vi "SpatialResolutionAnalysis-3D-8.vi"() -> ()   [LabVIEW 2024]
uses:
  <vilib>/Utility/miscctls.llb/LVBoundsTypeDef.ctl
  <vilib>/Utility/file.llb/Read Delimited Spreadsheet (DBL).vi
  <vilib>/picture/picture.llb/Draw True-Color Pixmap.vi
  <vilib>/gmath/NumericalOptimization/Nonlinear Curve Fit LM.vi
  <vilib>/regexp/Match Regular Expression.xnode
  <vilib>/Analysis/NI_AALBase.lvlib
  <vilib>/vision/NI_Vision_Development_Module.lvlib
  <vilib>/gmath/NI_Gmath.lvlib
panel:
  in  "saved parameter":dbl=15.0 format="%_6g"
  in  "save z pos?":bool
  in  "stop":bool
  in  "Range":cluster{"Lower value":sgl, "Upper value":sgl}={"Lower value"=302.0, "Upper value"=60055.0} {"Upper value" format="%.2f"; "Lower value" format="%.2f"}
  out "Numeric 3":i32=84
  out "profile 3":cluster{dbl[], dbl[]}[](graph)=[{[1.0, 1.0, 1.0, 1.0, 1.0, 1.0, 1.0, 1.0, 1.0, 1.0, 1.0, 1.0, 1.0, 2.0, 2.0, 2.0, 2.0, 2.0, 2.0, 2.0, 2.0, 2.0, 2.0, 2.0, 2.0, 2.0, 2.0, 2.0, 2.0, 2.0, 2.0, 5.0, 5.0, 5.0, 5.0, 5.0, 5.0, 5.0, 5.0, 5.0, 5.0, 5.0, 7.0, 7.0, 7.0, 7.0, 7.0, 7.0, 7.0, 7.0, 7.0, 7.0, 7.0, 7.0, 7.0, 7.0, 7.0, 7.0, 7.0, 7.0, 7.0, 3.0, 3.0, 3.0, 3.0, 3.0, 3.0, 3.0, 3.0, 3.0, 3.0, 1.0, 1.0, 15.0, 15.0, 15.0, 15.0, 15.0, 15.0, 15.0, 15.0, 15.0, 15.0, 15.0], [2.0133468228805937, 1.9830288608829862, 2.1410287615069046, 1.832229816874938, 1.7978233224426952, 1.968242110714196, 1.9933673041983153, 1.724601336050431, 2.5477060719979314, 1.9551201440941726, 1.8397170015620559, 2.236128582607133, 1.6264858204323749, 1.7869746298019815, 1.4196170843904827, 1.5374078182883288, 1.3782496628376637, 1.249895903925542, 1.3942037102048412, 1.4225030278735062, 1.433688545286691, 1.6920898620277007, 1.4435654626803172, 1.5101131998673663, 1.3060720728708268, 1.3178193530013447, 1.3649052519631513, 1.3097046992665182, 1.1134639493452403, 1.4424009490483098, 1.3428675394578506, 0.9421271973201978, 0.9192575100649564, 0.9861704571320219, 0.9992144079023442, 1.0853243609470147, 1.0439557604247962, 0.9041106621598265, 1.018147408083164, 1.1510621119284095, 1.115567444721871, 1.0954616791711456, 0.9694461946565243, 0.8684690878139703, 0.9376717749758984, 0.882216863445789, 1.1744088254801954, 0.9802461660244323, 0.997486368266876, 0.9419455677499634, 0.8628880149840508, 0.9268116414439239, 0.9181180722394033, 0.9776435525722661, 0.988995905088057, 0.9682008357747482, 0.9086257593875379, 1.040188271600828, 0.9299724706944195, 0.950388089905051, 0.9567309022594485, 1.221935897751796, 1.2090462045089128, 1.1438235149609108, 1.1493714387895813, 1.4345461597606564, 1.2239934520828633, 1.090228607115402, 1.354029262137178, 1.1569869611045591, 1.1967020722858934, 1.790272222951798, 1.6210900623548556, 1.0405059212935388, 1.0073358603798341, 0.9444257912585194, 0.9334882181118135, 0.9743355532381182, 0.8814598803657637, 0.8002331400158834, 0.8911247435086341, 0.8792614835678078, 0.921037700924059, 1.103404933894596]}, {[1.0, 1.0, 1.0, 1.0, 1.0, 1.0, 1.0, 1.0, 1.0, 1.0, 1.0, 1.0, 1.0, 2.0, 2.0, 2.0, 2.0, 2.0, 2.0, 2.0, 2.0, 2.0, 2.0, 2.0, 2.0, 2.0, 2.0, 2.0, 2.0, 2.0, 2.0, 5.0, 5.0, 5.0, 5.0, 5.0, 5.0, 5.0, 5.0, 5.0, 5.0, 5.0, 7.0, 7.0, 7.0, 7.0, 7.0, 7.0, 7.0, 7.0, 7.0, 7.0, 7.0, 7.0, 7.0, 7.0, 7.0, 7.0, 7.0, 7.0, 7.0, 3.0, 3.0, 3.0, 3.0, 3.0, 3.0, 3.0, 3.0, 3.0, 3.0, 1.0, 1.0, 15.0, 15.0, 15.0, 15.0, 15.0, 15.0, 15.0, 15.0, 15.0, 15.0, 15.0], [0.5349334014605461, 0.5381337297866883, 0.4325981122029295, 0.48916164520111804, 0.41556148299600454, 0.4850930072283453, 0.5673499365078756, 0.41714778173647393, 0.5526918869297825, 0.4923530041708235, 0.40501938702299484, 0.5082824398122024, 0.40354912909306634, 0.4530438324743144, 0.40779143741716084, 0.43077367983236237, 0.4671352516734954, 0.44629410664345487, 0.43158661278236216, 0.460271541886513, 0.4823249226541753, 0.5185727753496806, 0.4342974192886344, 0.45128050875740255, 0.4303885061603996, 0.5613218585443758, 0.41414445836126024, 0.44047765290288826, 0.47877243294417343, 0.46874740911159807, 0.4766614558480549, 0.4715857966455718, 0.4126072744806765, 0.42646841052591805, 0.40400976642452985, 0.4170504502787077, 0.48205219262233473, 0.41850180617403737, 0.41018388053645777, 0.44390188098962224, 0.41139907883701454, 0.4708303593503039, 0.4344403779325276, 0.46686047747542514, 0.48489083305355846, 0.4497629633492164, 0.46772433252337453, 0.4350416687080472, 0.40360520731331323, 0.4707299669639263, 0.38041949280922327, 0.4546761270737233, 0.44998728304625246, 0.48068592467547, 0.45909266188082487, 0.46566773053329674, 0.429218030475882, 0.41626874590441315, 0.4025480710092228, 0.46728163765248365, 0.46270168477314766, 0.47982606424071567, 0.40715128547570484, 0.4780994379451638, 0.40534745089527735, 0.44748638155411247, 0.49443443713902363, 0.44945698447630245, 0.46059272499696885, 0.43471888991751273, 0.4579720680900581, 0.43868811930073554, 0.4575463738995445, 0.45301271071412846, 0.4456849122856345, 0.44451647252412074, 0.46478062104722645, 0.40834206512347104, 0.46347713941761265, 0.4372934806506643, 0.4423639123216805, 0.4369146593472033, 0.4358778204397408, 0.4152090259272386]}, {[1.0, 1.0, 1.0, 1.0, 1.0, 1.0, 1.0, 1.0, 1.0, 1.0, 1.0, 1.0, 1.0, 2.0, 2.0, 2.0, 2.0, 2.0, 2.0, 2.0, 2.0, 2.0, 2.0, 2.0, 2.0, 2.0, 2.0, 2.0, 2.0, 2.0, 2.0, 5.0, 5.0, 5.0, 5.0, 5.0, 5.0, 5.0, 5.0, 5.0, 5.0, 5.0, 7.0, 7.0, 7.0, 7.0, 7.0, 7.0, 7.0, 7.0, 7.0, 7.0, 7.0, 7.0, 7.0, 7.0, 7.0, 7.0, 7.0, 7.0, 7.0, 3.0, 3.0, 3.0, 3.0, 3.0, 3.0, 3.0, 3.0, 3.0, 3.0, 1.0, 1.0, 15.0, 15.0, 15.0, 15.0, 15.0, 15.0, 15.0, 15.0, 15.0, 15.0, 15.0], [3.831063954171339, 3.059270830960583, 2.2982579267548897, 2.3512738574978624, 2.5538730276997903, 2.682560025330636, 2.6597875381449065, 2.7703141417989587, 3.0330629921976042, 2.546439917288072, 2.6225831316766848, 2.9353823913534747, 2.5991986482523224, 2.9173052067251684, 1.8789100817054876, 2.3734797215792143, 2.697188165514373, 2.0361242582660344, 2.698308173308555, 2.350622719228334, 2.1194094323864903, 2.83503408541773, 2.7683697804028498, 2.30213227302792, 2.8419209826307865, 2.1369921122360855, 2.009733489485215, 2.2188668846287496, 2.560644376786411, 2.0491758147172847, 2.29388213242103, 1.7032091300547687, 2.091295013582046, 1.8883702079287457, 1.5722793767576724, 1.497749085955476, 2.091931566369123, 1.804947152977885, 1.7777195448400112, 1.9539350987425426, 1.7816406998254182, 1.6103878576696868, 2.243284723289365, 1.439263985649626, 1.4421140948685303, 1.6012718104278727, 1.892588797177571, 1.8938395298902209, 1.663961362731013, 1.7664503089155017, 1.5923626379429023, 1.7924631613346518, 1.860054650973308, 1.8546487258879, 1.7533530517676261, 1.6570807100677052, 1.7721806371618676, 1.860204996421116, 1.9831442631444507, 1.7905475389437313, 1.8278060844960526, 2.14740251637709, 1.6527221427498724, 2.2734081810795557, 1.7682142456430505, 2.351440748167282, 2.039692073403972, 2.249697494044236, 2.019669976655679, 2.3817391436774127, 2.1044693016718634, 2.945123441454935, 3.132984030089959, 1.4322347170702565, 1.8617388862479958, 1.7668984450954066, 1.9239338358912674, 1.7440910356590962, 1.8497936230767198, 1.9984535114889663, 1.9016492433228582, 1.8183778696194395, 1.756109772929477, 1.864696210002186]}, {[1.0, 1.0, 1.0, 1.0, 1.0, 1.0, 1.0, 1.0, 1.0, 1.0, 1.0, 1.0, 1.0, 2.0, 2.0, 2.0, 2.0, 2.0, 2.0, 2.0, 2.0, 2.0, 2.0, 2.0, 2.0, 2.0, 2.0, 2.0, 2.0, 2.0, 2.0, 5.0, 5.0, 5.0, 5.0, 5.0, 5.0, 5.0, 5.0, 5.0, 5.0, 5.0, 7.0, 7.0, 7.0, 7.0, 7.0, 7.0, 7.0, 7.0, 7.0, 7.0, 7.0, 7.0, 7.0, 7.0, 7.0, 7.0, 7.0, 7.0, 7.0, 3.0, 3.0, 3.0, 3.0, 3.0, 3.0, 3.0, 3.0, 3.0, 3.0, 1.0, 1.0, 15.0, 15.0, 15.0, 15.0, 15.0, 15.0, 15.0, 15.0, 15.0, 15.0, 15.0], [2.1950609171334663, 2.054618641938806, 2.104623270933475, 2.175230158941747, 1.8063966644943987, 2.1295671490810504, 2.209023498381645, 2.0515957222532695, 2.9990312250832534, 2.2759668684117713, 2.281844375004091, 2.4517643206281377, 0.9998405968995983, 1.9895569035078806, 1.386277332900748, 1.477211472520211, 1.4491295731261742, 1.295484538599624, 1.2209490171797608, 1.328049693706136, 1.3871687988938963, 1.6950226848823489, 1.3919183622385123, 1.530122363720778, 1.4218506232848938, 1.814696520405228, 1.499546890762415, 1.3528630093363747, 1.1830279345524057, 1.4487275307919036, 1.3903221708836062, 0.9299541953106812, 0.8839351063390566, 1.035489598307442, 1.009482788308503, 1.054044052714303, 1.0236198842257271, 1.0318268251460063, 1.1225026575045192, 1.167009429834893, 0.9257403035306736, 1.070234933121553, 0.9920706919584273, 0.9140544351981513, 0.8757808606546661, 0.8718346074707618, 1.0110444436389308, 0.9520818427957021, 0.9768177701203681, 0.9915186544650038, 0.9230083868636685, 0.9046033708789486, 0.9099211724070002, 1.002151816664439, 0.9608485679370016, 0.9125676936610334, 0.9660386410221703, 1.078401400423473, 1.0023703508557482, 0.895286648365859, 0.9716597443982098, 1.1949613429126829, 1.161748827048745, 1.1631282077159188, 1.148313006075648, 1.3735217290054094, 1.2433597954356586, 1.1662345174848958, 1.2701690085899722, 1.1727390746235637, 1.1971761228612998, 2.0031359293798054, 2.0609983678438337, 0.9149174421733332, 1.0525064576834762, 0.9347056385035375, 0.946629434078085, 1.5404013619903427, 0.930605986788623, 0.9051875232044269, 0.894279488961371, 0.8718853102409165, 0.9292096538995072, 1.0776975442315762]}, {[1.0, 1.0, 1.0, 1.0, 1.0, 1.0, 1.0, 1.0, 1.0, 1.0, 1.0, 1.0, 1.0, 2.0, 2.0, 2.0, 2.0, 2.0, 2.0, 2.0, 2.0, 2.0, 2.0, 2.0, 2.0, 2.0, 2.0, 2.0, 2.0, 2.0, 2.0, 5.0, 5.0, 5.0, 5.0, 5.0, 5.0, 5.0, 5.0, 5.0, 5.0, 5.0, 7.0, 7.0, 7.0, 7.0, 7.0, 7.0, 7.0, 7.0, 7.0, 7.0, 7.0, 7.0, 7.0, 7.0, 7.0, 7.0, 7.0, 7.0, 7.0, 3.0, 3.0, 3.0, 3.0, 3.0, 3.0, 3.0, 3.0, 3.0, 3.0, 1.0, 1.0, 15.0, 15.0, 15.0, 15.0, 15.0, 15.0, 15.0, 15.0, 15.0, 15.0, 15.0], [2.9152156827594293, 2.5990526581184956, 1.906401812221069, 2.3686457243679144, 2.121321629827777, 2.3179713514009026, 2.392123629004429, 2.3037200675462755, 2.9146261263558007, 2.0648914087567856, 2.484756888015519, 2.4235500991471604, 1.533300131698492, 2.500295338025416, 2.3348778310327094, 2.405355608068957, 2.528663329870978, 2.2469147380725674, 2.4434672372828383, 2.1118260376977456, 2.721672790630798, 3.1052449674871614, 2.7801574803549274, 2.627964587450267, 2.474809806384693, 1.7158461369035183, 2.1448277490061587, 2.0290842777452047, 2.463419621353616, 3.5693252371416606, 2.5104117383774973, 2.241237982322342, 1.7078526466721193, 2.0495685256164693, 1.7370219820601127, 1.8245896378450086, 2.5086646334752323, 2.1859796911332667, 2.180925068929074, 2.012040182338204, 2.273553445872903, 1.949240216124691, 2.5350823425047007, 1.573081961156342, 1.867172753412812, 2.141389794448718, 2.0778586256984615, 2.0938614883880526, 2.101194097948842, 1.992923549444901, 1.7936881545636807, 1.9749097104449778, 2.045208462819868, 2.2293085556006202, 2.2248086215455687, 2.1608335627654767, 2.262287525483442, 2.2543964739278, 2.0932173803022063, 2.0184068032417786, 2.150789163948129, 2.2053407496814255, 2.106580809562779, 2.0176046290868026, 2.104550211229832, 2.4659027742456647, 2.2702529865700116, 2.284568939068995, 2.2528486161897474, 2.268035269102454, 2.2830606744651365, 2.8430238588896906, 2.8219479955311835, 1.7946822327277403, 2.334201107146507, 2.032573581439689, 2.183270787877003, 2.124268915381388, 1.9879932478731197, 2.344731423243975, 2.0123274416218733, 2.215117623104961, 2.2701610476768646, 2.247837372716093]}]
  out "Image":T1(plugin-control)
  out "obj index":i32
  in  "analysis file":path=path "E:/PSFvsR.anal"
  in  "delete":bool
  in  "add":bool
  in  "stocked object index":i32(slide) min=0 max=2 scale=0.0..2.0
  in  "stocked / raw":bool=TRUE
  out "FWHMx'":dbl=1.1390586789611326
  out "FWHMz'":dbl=2.7153633068041123
  out "x'":cluster{dbl[], dbl[]}[](graph)=[{[-2.1729316492173996, -1.9681427393245199, -1.7633538294316402, -1.5585649195387605, -1.353776009645881, -1.1489870997530014, -0.9441981898601217, -0.739409279967242, -0.5346203700743624, -0.32983146018148274, -0.1250425502886031, 0.07974635960427658, 0.28453526949715624, 0.48932417939003586, 0.6941130892829155, 0.8989019991757952, 1.1036909090686748, 1.3084798189615545, 1.5132687288544342, 1.7180576387473139, 1.9228465486401933], [49.0, 26.0, 15.0, 15.0, 19.0, 38.0, 88.0, 186.0, 324.0, 487.0, 578.0, 545.0, 450.0, 335.0, 242.0, 169.0, 120.0, 87.0, 69.0, 57.0, 47.0]}, {array[1000 elements], array[1000 elements]}]
  out "z'":cluster{dbl[], dbl[]}[](graph)=[{[-2.9476850843070337, -2.742896174414154, -2.5381072645212743, -2.333318354628395, -2.128529444735515, -1.9237405348426353, -1.7189516249497558, -1.5141627150568762, -1.3093738051639965, -1.1045848952711168, -0.8997959853782371, -0.6950070754853575, -0.49021816559247783, -0.2854292556995982, -0.08064034580671856, 0.1241485640861611, 0.3289374739790408, 0.5337263838719204, 0.7385152937648001, 0.9433042036576798, 1.1480931135505594, 1.352882023443439, 1.5576709333363186, 1.7624598432291982, 1.967248753122078, 2.1720376630149576, 2.376826572907837], [33.0, 39.0, 53.0, 72.0, 93.0, 128.0, 182.0, 228.0, 282.0, 342.0, 407.0, 503.0, 557.0, 578.0, 538.0, 507.0, 494.0, 456.0, 415.0, 378.0, 329.0, 274.0, 240.0, 223.0, 188.0, 156.0, 130.0]}, {array[1000 elements], array[1000 elements]}]
  in  "Angle (degrees)":dbl=-23.0 format="%.2f"
  in  "nx'":i32=10
  in  "nz'":i32=13
  out "zx 2":u16[][](graph)=[[0, 0, 0, 0, 0, 0, 214, 195, 168, 154, 142, 125, 111, 106, 109, 112, 114, 112, 109, 111, 116, 122, 126, 126, 124, 124, 134, 0, 0, 0, 0, 0, 0, 0, 0, 0, 0, 0, 0, 0], [0, 0, 0, 0, 0, 0, 234, 188, 163, 151, 142, 128, 115, 115, 114, 113, 112, 112, 112, 113, 119, 125, 127, 126, 128, 133, 135, 134, 127, 0, 0, 0, 0, 0, 0, 0, 0, 0, 0, 0], [0, 0, 0, 0, 0, 246, 230, 176, 154, 145, 128, 122, 119, 118, 117, 115, 113, 113, 116, 117, 121, 128, 130, 135, 146, 153, 152, 138, 125, 122, 124, 0, 0, 0, 0, 0, 0, 0, 0, 0], [0, 0, 0, 0, 0, 215, 201, 171, 153, 138, 128, 123, 121, 120, 118, 115, 114, 112, 111, 118, 125, 132, 138, 153, 168, 169, 153, 141, 131, 128, 126, 117, 113, 114, 0, 0, 0, 0, 0, 0], [0, 0, 0, 0, 257, 240, 191, 168, 146, 132, 128, 126, 124, 122, 118, 116, 115, 113, 112, 121, 131, 133, 145, 162, 170, 162, 150, 142, 137, 136, 133, 119, 114, 116, 111, 105, 0, 0, 0, 0], [0, 0, 0, 0, 279, 243, 192, 163, 140, 126, 125, 126, 123, 119, 116, 116, 115, 117, 122, 127, 134, 139, 148, 164, 171, 161, 155, 149, 149, 145, 135, 123, 119, 118, 114, 104, 106, 108, 0, 0], [0, 0, 0, 274, 280, 223, 182, 157, 136, 124, 121, 122, 119, 116, 114, 114, 114, 122, 133, 138, 146, 153, 160, 171, 179, 177, 165, 155, 155, 148, 135, 129, 128, 127, 121, 113, 109, 108, 105, 104], [0, 0, 0, 259, 246, 198, 164, 150, 138, 132, 128, 123, 119, 116, 116, 116, 115, 121, 135, 149, 162, 172, 182, 181, 190, 191, 177, 164, 158, 148, 139, 135, 133, 127, 121, 115, 112, 111, 107, 106], [0, 0, 0, 243, 225, 184, 157, 148, 143, 141, 138, 127, 117, 117, 115, 117, 118, 123, 130, 146, 169, 193, 206, 207, 208, 206, 187, 177, 168, 155, 143, 137, 128, 120, 115, 113, 112, 113, 108, 109], [0, 0, 217, 224, 214, 179, 167, 157, 147, 148, 147, 137, 126, 118, 114, 114, 117, 124, 128, 155, 195, 228, 243, 250, 242, 221, 198, 185, 176, 162, 146, 135, 124, 118, 113, 109, 111, 113, 113, 114], [0, 0, 190, 203, 199, 187, 176, 164, 155, 160, 159, 150, 134, 118, 112, 110, 112, 124, 147, 186, 238, 282, 295, 294, 271, 239, 207, 190, 181, 169, 150, 133, 126, 122, 114, 111, 112, 115, 116, 115], [0, 161, 169, 188, 185, 190, 186, 173, 164, 166, 166, 157, 135, 116, 113, 112, 114, 135, 168, 216, 279, 328, 340, 325, 292, 251, 216, 193, 187, 174, 150, 135, 129, 124, 117, 116, 118, 119, 118, 115], [0, 149, 162, 174, 176, 184, 188, 178, 170, 166, 168, 157, 132, 113, 111, 116, 125, 147, 188, 250, 327, 382, 388, 354, 303, 259, 221, 206, 198, 181, 154, 139, 131, 126, 123, 120, 121, 122, 119, 116], [133, 137, 156, 167, 169, 179, 187, 183, 176, 174, 173, 160, 134, 118, 113, 116, 128, 157, 216, 298, 384, 442, 441, 390, 329, 282, 248, 226, 207, 184, 163, 149, 137, 133, 130, 126, 126, 125, 119, 119], [127, 132, 145, 157, 162, 177, 196, 190, 181, 183, 183, 166, 141, 124, 117, 119, 133, 166, 238, 337, 442, 507, 506, 449, 373, 315, 276, 236, 204, 181, 164, 151, 140, 137, 133, 131, 132, 126, 118, 113], [123, 126, 137, 146, 155, 172, 193, 191, 178, 184, 193, 169, 140, 124, 119, 123, 141, 182, 257, 373, 509, 603, 578, 496, 403, 326, 276, 234, 198, 174, 158, 145, 139, 137, 134, 131, 129, 122, 115, 112], [117, 122, 132, 139, 149, 175, 185, 177, 173, 180, 183, 163, 133, 115, 116, 122, 138, 185, 264, 407, 574, 657, 617, 527, 427, 333, 267, 223, 189, 170, 153, 143, 138, 135, 132, 125, 121, 120, 118, 115], [118, 121, 125, 132, 146, 166, 175, 166, 163, 174, 171, 149, 126, 115, 115, 119, 138, 188, 286, 424, 587, 678, 645, 550, 435, 342, 269, 220, 187, 169, 157, 147, 138, 132, 127, 121, 122, 124, 121, 116], [122, 120, 121, 129, 139, 152, 159, 157, 158, 164, 157, 135, 120, 117, 120, 123, 143, 201, 298, 422, 550, 638, 631, 536, 420, 337, 276, 221, 186, 165, 157, 148, 137, 129, 125, 125, 129, 131, 124, 117], [125, 123, 122, 128, 133, 142, 147, 146, 153, 156, 143, 124, 112, 115, 116, 123, 143, 186, 284, 408, 536, 607, 594, 512, 416, 336, 271, 219, 183, 158, 145, 142, 137, 131, 129, 134, 138, 135, 127, 123], [126, 123, 123, 128, 140, 147, 146, 141, 146, 141, 140, 126, 116, 114, 117, 127, 145, 185, 270, 389, 517, 594, 577, 503, 406, 316, 251, 206, 177, 157, 142, 135, 130, 127, 130, 134, 139, 136, 133, 132], [123, 120, 120, 126, 139, 145, 147, 144, 147, 151, 144, 129, 117, 117, 123, 133, 149, 189, 267, 373, 488, 556, 553, 484, 384, 291, 229, 189, 169, 155, 140, 130, 123, 124, 128, 135, 138, 139, 141, 140], [121, 122, 123, 121, 125, 135, 136, 138, 147, 148, 139, 125, 118, 121, 127, 137, 154, 192, 255, 357, 464, 515, 504, 442, 348, 272, 215, 180, 163, 152, 138, 127, 123, 127, 137, 141, 143, 149, 151, 148], [121, 124, 126, 123, 125, 132, 134, 135, 138, 135, 129, 119, 119, 124, 127, 137, 151, 180, 235, 328, 428, 478, 465, 415, 337, 262, 203, 177, 160, 147, 136, 129, 129, 137, 147, 147, 151, 159, 159, 153], [121, 123, 126, 123, 124, 130, 133, 134, 132, 130, 125, 122, 122, 123, 123, 134, 148, 173, 223, 304, 383, 429, 430, 390, 317, 242, 195, 173, 155, 142, 137, 132, 136, 141, 143, 146, 153, 158, 159, 154], [126, 130, 131, 129, 127, 129, 133, 133, 128, 129, 127, 121, 121, 122, 130, 140, 152, 173, 211, 268, 332, 374, 393, 359, 285, 216, 180, 161, 148, 140, 139, 136, 136, 138, 138, 144, 152, 164, 165, 163], [131, 136, 134, 130, 128, 132, 136, 128, 120, 124, 124, 120, 121, 125, 137, 146, 154, 168, 194, 235, 289, 340, 367, 342, 273, 198, 157, 147, 141, 140, 140, 137, 135, 136, 140, 151, 169, 179, 174, 172], [124, 127, 128, 128, 130, 133, 135, 126, 120, 123, 120, 118, 121, 127, 137, 145, 151, 162, 180, 213, 270, 323, 349, 337, 268, 197, 156, 143, 136, 138, 141, 141, 137, 135, 143, 163, 182, 184, 178, 0], [116, 122, 127, 132, 133, 134, 134, 129, 126, 126, 124, 122, 125, 131, 141, 149, 154, 156, 168, 204, 250, 288, 309, 314, 250, 190, 160, 145, 134, 134, 138, 139, 135, 139, 149, 170, 184, 185, 185, 0], [117, 120, 126, 135, 131, 135, 137, 135, 132, 130, 129, 128, 133, 142, 149, 157, 159, 154, 163, 193, 230, 256, 267, 258, 221, 181, 160, 144, 131, 125, 130, 130, 129, 135, 150, 165, 177, 183, 0, 0], [118, 119, 123, 129, 130, 135, 140, 139, 136, 134, 130, 129, 135, 142, 148, 153, 154, 150, 155, 177, 208, 230, 244, 226, 199, 175, 158, 140, 130, 124, 125, 126, 127, 137, 150, 167, 186, 184, 0, 0], [118, 122, 126, 124, 130, 138, 139, 135, 135, 135, 126, 125, 134, 142, 142, 144, 146, 141, 146, 165, 187, 208, 225, 218, 200, 177, 150, 139, 131, 126, 124, 124, 128, 137, 154, 181, 198, 0, 0, 0], [108, 117, 118, 120, 128, 138, 136, 132, 132, 130, 125, 124, 132, 138, 141, 141, 140, 135, 141, 157, 172, 186, 203, 207, 190, 161, 143, 135, 129, 125, 125, 123, 126, 139, 160, 185, 197, 0, 0, 0], [105, 109, 113, 117, 125, 130, 131, 129, 129, 128, 123, 118, 123, 133, 138, 136, 133, 128, 133, 144, 159, 173, 189, 200, 180, 149, 140, 136, 130, 128, 131, 133, 138, 148, 164, 178, 185, 0, 0, 0], [0, 0, 113, 110, 101, 117, 120, 122, 123, 121, 116, 113, 119, 130, 134, 126, 126, 124, 124, 139, 155, 167, 180, 188, 175, 151, 142, 138, 133, 136, 141, 143, 146, 149, 161, 170, 0, 0, 0, 0], [0, 0, 0, 0, 101, 110, 106, 116, 120, 116, 110, 110, 116, 122, 120, 117, 120, 121, 121, 134, 148, 159, 169, 178, 168, 153, 145, 142, 141, 144, 147, 142, 146, 151, 164, 167, 0, 0, 0, 0], [0, 0, 0, 0, 0, 0, 109, 116, 118, 113, 109, 105, 110, 112, 110, 110, 114, 116, 119, 128, 140, 152, 160, 165, 159, 152, 148, 143, 148, 154, 149, 144, 145, 153, 164, 0, 0, 0, 0, 0], [0, 0, 0, 0, 0, 0, 0, 0, 0, 111, 108, 107, 105, 106, 106, 109, 112, 110, 113, 123, 135, 145, 150, 152, 152, 152, 151, 151, 152, 152, 148, 144, 142, 151, 154, 0, 0, 0, 0, 0], [0, 0, 0, 0, 0, 0, 0, 0, 0, 0, 0, 108, 96, 95, 102, 109, 110, 109, 113, 123, 132, 137, 137, 138, 147, 158, 165, 163, 160, 160, 153, 146, 145, 153, 0, 0, 0, 0, 0, 0], [0, 0, 0, 0, 0, 0, 0, 0, 0, 0, 0, 0, 0, 96, 103, 110, 111, 111, 116, 120, 125, 126, 127, 132, 146, 164, 174, 169, 166, 169, 164, 151, 148, 153, 0, 0, 0, 0, 0, 0]]
  out "num of points":i32=3
  out "profile 2":cluster{dbl[], dbl[]}[](graph)=[{[15.0, 15.0, 15.0], [0.8792614835678078, 0.921037700924059, 1.103404933894596]}, {[15.0, 15.0, 15.0], [0.4369146593472033, 0.4358778204397408, 0.4152090259272386]}, {[15.0, 15.0, 15.0], [1.8183778696194395, 1.756109772929477, 1.864696210002186]}, {[15.0, 15.0, 15.0], [0.8718853102409165, 0.9292096538995072, 1.0776975442315762]}, {[15.0, 15.0, 15.0], [2.215117623104961, 2.2701610476768646, 2.247837372716093]}]
  out "z [um]":dbl=0.23987999999999998
  out "Nx":i32=109
  out "Ny":i32=57
  out "Nz":i32=40
  out "z ofst and pixsize":dbl[](array[numeric])=[0.57912, 0.20475]
  in  "most recent":bool=TRUE
  in  "folderpath":path=path "E:/20241006-215727beads"
  out "Numeric 2":i32=2402
  in  "fitting range y":dbl=8.0
  in  "fitting range z":dbl=30.0
  out "Particle Reports (Pixels)":T2(array[cluster])=[{"Area"=37.0, "Number of Holes"=0.0, "Bounding Rect"={"Left"=52.0, "Top"=2.0, "Right"=63.0, "Bottom"=7.0}, "Center of Mass"={"X"=57.16216216216216, "Y"=3.6216216216216215}, "Orientation"=179.34423482631453, "Dimensions"={"Width"=11.0, "Height"=5.0}}, {"Area"=30.0, "Number of Holes"=0.0, "Bounding Rect"={"Left"=29.0, "Top"=4.0, "Right"=44.0, "Bottom"=9.0}, "Center of Mass"={"X"=36.166666666666664, "Y"=5.733333333333333}, "Orientation"=165.68755166285754, "Dimensions"={"Width"=15.0, "Height"=5.0}}, {"Area"=8.0, "Number of Holes"=0.0, "Bounding Rect"={"Left"=76.0, "Top"=5.0, "Right"=81.0, "Bottom"=7.0}, "Center of Mass"={"X"=78.0, "Y"=5.625}, "Orientation"=-0.0, "Dimensions"={"Width"=5.0, "Height"=2.0}}, {"Area"=6.0, "Number of Holes"=0.0, "Bounding Rect"={"Left"=90.0, "Top"=5.0, "Right"=94.0, "Bottom"=7.0}, "Center of Mass"={"X"=91.5, "Y"=5.333333333333333}, "Orientation"=-0.0, "Dimensions"={"Width"=4.0, "Height"=2.0}}, {"Area"=1.0, "Number of Holes"=0.0, "Bounding Rect"={"Left"=22.0, "Top"=6.0, "Right"=23.0, "Bottom"=7.0}, "Center of Mass"={"X"=22.0, "Y"=6.0}, "Orientation"=-0.0, "Dimensions"={"Width"=1.0, "Height"=1.0}}, {"Area"=9.0, "Number of Holes"=0.0, "Bounding Rect"={"Left"=67.0, "Top"=6.0, "Right"=72.0, "Bottom"=9.0}, "Center of Mass"={"X"=69.33333333333333, "Y"=7.222222222222222}, "Orientation"=167.962250872462, "Dimensions"={"Width"=5.0, "Height"=3.0}}, {"Area"=10.0, "Number of Holes"=0.0, "Bounding Rect"={"Left"=82.0, "Top"=11.0, "Right"=87.0, "Bottom"=13.0}, "Center of Mass"={"X"=84.0, "Y"=11.5}, "Orientation"=-0.0, "Dimensions"={"Width"=5.0, "Height"=2.0}}, {"Area"=7.0, "Number of Holes"=0.0, "Bounding Rect"={"Left"=92.0, "Top"=11.0, "Right"=97.0, "Bottom"=13.0}, "Center of Mass"={"X"=94.14285714285714, "Y"=11.285714285714286}, "Orientation"=175.69217590792118, "Dimensions"={"Width"=5.0, "Height"=2.0}}, {"Area"=6.0, "Number of Holes"=0.0, "Bounding Rect"={"Left"=65.0, "Top"=13.0, "Right"=69.0, "Bottom"=15.0}, "Center of Mass"={"X"=66.83333333333333, "Y"=13.333333333333334}, "Orientation"=167.06682160295298, "Dimensions"={"Width"=4.0, "Height"=2.0}}, {"Area"=7.0, "Number of Holes"=0.0, "Bounding Rect"={"Left"=73.0, "Top"=13.0, "Right"=77.0, "Bottom"=15.0}, "Center of Mass"={"X"=74.28571428571429, "Y"=13.571428571428571}, "Orientation"=171.65037788300214, "Dimensions"={"Width"=4.0, "Height"=2.0}}, {"Area"=24.0, "Number of Holes"=0.0, "Bounding Rect"={"Left"=22.0, "Top"=14.0, "Right"=32.0, "Bottom"=18.0}, "Center of Mass"={"X"=27.0, "Y"=15.625}, "Orientation"=14.883749397417526, "Dimensions"={"Width"=10.0, "Height"=4.0}}, {"Area"=24.0, "Number of Holes"=0.0, "Bounding Rect"={"Left"=48.0, "Top"=15.0, "Right"=55.0, "Bottom"=21.0}, "Center of Mass"={"X"=51.041666666666664, "Y"=17.541666666666668}, "Orientation"=140.81219786217568, "Dimensions"={"Width"=7.0, "Height"=6.0}}, {"Area"=15.0, "Number of Holes"=0.0, "Bounding Rect"={"Left"=10.0, "Top"=19.0, "Right"=15.0, "Bottom"=23.0}, "Center of Mass"={"X"=12.333333333333334, "Y"=20.266666666666666}, "Orientation"=174.11585553399107, "Dimensions"={"Width"=5.0, "Height"=4.0}}, {"Area"=8.0, "Number of Holes"=0.0, "Bounding Rect"={"Left"=29.0, "Top"=20.0, "Right"=34.0, "Bottom"=23.0}, "Center of Mass"={"X"=31.25, "Y"=21.125}, "Orientation"=164.64358614242056, "Dimensions"={"Width"=5.0, "Height"=3.0}}, {"Area"=6.0, "Number of Holes"=0.0, "Bounding Rect"={"Left"=77.0, "Top"=21.0, "Right"=81.0, "Bottom"=23.0}, "Center of Mass"={"X"=78.5, "Y"=21.333333333333332}, "Orientation"=-0.0, "Dimensions"={"Width"=4.0, "Height"=2.0}}, {"Area"=12.0, "Number of Holes"=0.0, "Bounding Rect"={"Left"=26.0, "Top"=25.0, "Right"=30.0, "Bottom"=30.0}, "Center of Mass"={"X"=27.833333333333332, "Y"=26.833333333333332}, "Orientation"=69.54280838998545, "Dimensions"={"Width"=4.0, "Height"=5.0}}, {"Area"=3.0, "Number of Holes"=0.0, "Bounding Rect"={"Left"=70.0, "Top"=26.0, "Right"=73.0, "Bottom"=27.0}, "Center of Mass"={"X"=71.0, "Y"=26.0}, "Orientation"=-0.0, "Dimensions"={"Width"=3.0, "Height"=1.0}}, {"Area"=7.0, "Number of Holes"=0.0, "Bounding Rect"={"Left"=4.0, "Top"=28.0, "Right"=8.0, "Bottom"=30.0}, "Center of Mass"={"X"=5.714285714285714, "Y"=28.428571428571427}, "Orientation"=171.65037788300342, "Dimensions"={"Width"=4.0, "Height"=2.0}}, {"Area"=5.0, "Number of Holes"=0.0, "Bounding Rect"={"Left"=83.0, "Top"=28.0, "Right"=86.0, "Bottom"=30.0}, "Center of Mass"={"X"=84.2, "Y"=28.4}, "Orientation"=161.56505117709622, "Dimensions"={"Width"=3.0, "Height"=2.0}}, {"Area"=9.0, "Number of Holes"=0.0, "Bounding Rect"={"Left"=89.0, "Top"=28.0, "Right"=94.0, "Bottom"=30.0}, "Center of Mass"={"X"=91.22222222222223, "Y"=28.444444444444443}, "Orientation"=175.26883889599605, "Dimensions"={"Width"=5.0, "Height"=2.0}}, {"Area"=7.0, "Number of Holes"=0.0, "Bounding Rect"={"Left"=52.0, "Top"=29.0, "Right"=57.0, "Bottom"=31.0}, "Center of Mass"={"X"=53.857142857142854, "Y"=29.714285714285715}, "Orientation"=175.6921759079141, "Dimensions"={"Width"=5.0, "Height"=2.0}}, {"Area"=7.0, "Number of Holes"=0.0, "Bounding Rect"={"Left"=65.0, "Top"=29.0, "Right"=69.0, "Bottom"=31.0}, "Center of Mass"={"X"=66.71428571428571, "Y"=29.428571428571427}, "Orientation"=171.65037788300276, "Dimensions"={"Width"=4.0, "Height"=2.0}}, {"Area"=1.0, "Number of Holes"=0.0, "Bounding Rect"={"Left"=96.0, "Top"=29.0, "Right"=97.0, "Bottom"=30.0}, "Center of Mass"={"X"=96.0, "Y"=29.0}, "Orientation"=-0.0, "Dimensions"={"Width"=1.0, "Height"=1.0}}, {"Area"=25.0, "Number of Holes"=0.0, "Bounding Rect"={"Left"=3.0, "Top"=33.0, "Right"=9.0, "Bottom"=38.0}, "Center of Mass"={"X"=5.4, "Y"=34.96}, "Orientation"=10.870389527236576, "Dimensions"={"Width"=6.0, "Height"=5.0}}, {"Area"=16.0, "Number of Holes"=0.0, "Bounding Rect"={"Left"=59.0, "Top"=33.0, "Right"=65.0, "Bottom"=36.0}, "Center of Mass"={"X"=61.75, "Y"=33.875}, "Orientation"=172.42714692778492, "Dimensions"={"Width"=6.0, "Height"=3.0}}, {"Area"=1.0, "Number of Holes"=0.0, "Bounding Rect"={"Left"=25.0, "Top"=34.0, "Right"=26.0, "Bottom"=35.0}, "Center of Mass"={"X"=25.0, "Y"=34.0}, "Orientation"=-0.0, "Dimensions"={"Width"=1.0, "Height"=1.0}}, {"Area"=9.0, "Number of Holes"=0.0, "Bounding Rect"={"Left"=39.0, "Top"=40.0, "Right"=44.0, "Bottom"=42.0}, "Center of Mass"={"X"=41.22222222222222, "Y"=40.44444444444444}, "Orientation"=175.26883889598594, "Dimensions"={"Width"=5.0, "Height"=2.0}}, {"Area"=1.0, "Number of Holes"=0.0, "Bounding Rect"={"Left"=73.0, "Top"=42.0, "Right"=74.0, "Bottom"=43.0}, "Center of Mass"={"X"=73.0, "Y"=42.0}, "Orientation"=-0.0, "Dimensions"={"Width"=1.0, "Height"=1.0}}, {"Area"=8.0, "Number of Holes"=0.0, "Bounding Rect"={"Left"=35.0, "Top"=43.0, "Right"=39.0, "Bottom"=45.0}, "Center of Mass"={"X"=36.5, "Y"=43.5}, "Orientation"=-0.0, "Dimensions"={"Width"=4.0, "Height"=2.0}}, {"Area"=8.0, "Number of Holes"=0.0, "Bounding Rect"={"Left"=30.0, "Top"=44.0, "Right"=34.0, "Bottom"=46.0}, "Center of Mass"={"X"=31.5, "Y"=44.5}, "Orientation"=-0.0, "Dimensions"={"Width"=4.0, "Height"=2.0}}, {"Area"=2.0, "Number of Holes"=0.0, "Bounding Rect"={"Left"=53.0, "Top"=44.0, "Right"=55.0, "Bottom"=45.0}, "Center of Mass"={"X"=53.5, "Y"=44.0}, "Orientation"=-0.0, "Dimensions"={"Width"=2.0, "Height"=1.0}}, {"Area"=36.0, "Number of Holes"=0.0, "Bounding Rect"={"Left"=36.0, "Top"=46.0, "Right"=47.0, "Bottom"=51.0}, "Center of Mass"={"X"=40.52777777777778, "Y"=47.77777777777778}, "Orientation"=171.22278809294195, "Dimensions"={"Width"=11.0, "Height"=5.0}}, {"Area"=5.0, "Number of Holes"=0.0, "Bounding Rect"={"Left"=88.0, "Top"=46.0, "Right"=91.0, "Bottom"=48.0}, "Center of Mass"={"X"=89.2, "Y"=46.6}, "Orientation"=18.4349488228699, "Dimensions"={"Width"=3.0, "Height"=2.0}}, {"Area"=8.0, "Number of Holes"=0.0, "Bounding Rect"={"Left"=74.0, "Top"=48.0, "Right"=79.0, "Bottom"=51.0}, "Center of Mass"={"X"=76.5, "Y"=48.875}, "Orientation"=7.545786339297439, "Dimensions"={"Width"=5.0, "Height"=3.0}}, {"Area"=3.0, "Number of Holes"=0.0, "Bounding Rect"={"Left"=48.0, "Top"=50.0, "Right"=51.0, "Bottom"=51.0}, "Center of Mass"={"X"=49.0, "Y"=50.0}, "Orientation"=-0.0, "Dimensions"={"Width"=3.0, "Height"=1.0}}, {"Area"=30.0, "Number of Holes"=0.0, "Bounding Rect"={"Left"=66.0, "Top"=51.0, "Right"=77.0, "Bottom"=55.0}, "Center of Mass"={"X"=71.83333333333333, "Y"=52.833333333333336}, "Orientation"=4.05699723021086, "Dimensions"={"Width"=11.0, "Height"=4.0}}, {"Area"=4.0, "Number of Holes"=0.0, "Bounding Rect"={"Left"=83.0, "Top"=52.0, "Right"=86.0, "Bottom"=54.0}, "Center of Mass"={"X"=84.0, "Y"=52.25}, "Orientation"=-0.0, "Dimensions"={"Width"=3.0, "Height"=2.0}}, {"Area"=4.0, "Number of Holes"=0.0, "Bounding Rect"={"Left"=35.0, "Top"=54.0, "Right"=39.0, "Bottom"=55.0}, "Center of Mass"={"X"=36.5, "Y"=54.0}, "Orientation"=-0.0, "Dimensions"={"Width"=4.0, "Height"=1.0}}, {"Area"=2.0, "Number of Holes"=0.0, "Bounding Rect"={"Left"=99.0, "Top"=55.0, "Right"=101.0, "Bottom"=56.0}, "Center of Mass"={"X"=99.5, "Y"=55.0}, "Orientation"=-0.0, "Dimensions"={"Width"=2.0, "Height"=1.0}}]
  out "error z":dbl=0.6513882337485863
  out "error y":dbl=3.612958681902941
  out "error x":dbl=1.7215369706106136
  out "file path (use dialog)":path=path "E:/20241006-215727beads/20241006-215727beadsaiviatif/20241006-215727beads_t0.aivia.tif"
  out "yx 5":u16[][](graph)=[[135, 135, 135, 135, 135, 135, 135, 135, 135, 135, 135, 135, 135, 135, 135, 135, 135, 135, 135, 135], [135, 135, 135, 135, 135, 135, 135, 135, 135, 136, 135, 135, 135, 135, 135, 135, 135, 135, 135, 135], [135, 135, 135, 135, 135, 135, 135, 135, 136, 138, 138, 138, 136, 135, 135, 135, 135, 135, 135, 135], [135, 135, 135, 135, 135, 135, 135, 136, 139, 143, 145, 142, 138, 136, 135, 135, 135, 135, 135, 135], [135, 135, 135, 135, 135, 135, 135, 138, 145, 155, 160, 154, 144, 138, 135, 135, 135, 135, 135, 135], [135, 135, 135, 135, 135, 135, 135, 141, 156, 177, 186, 174, 154, 141, 136, 135, 135, 135, 135, 135], [135, 135, 135, 135, 135, 135, 136, 146, 173, 211, 228, 207, 169, 145, 137, 135, 135, 135, 135, 135], [135, 135, 135, 135, 135, 135, 138, 153, 197, 258, 287, 252, 190, 151, 138, 135, 135, 135, 135, 135], [135, 135, 135, 135, 135, 135, 139, 161, 222, 313, 355, 302, 214, 157, 139, 135, 135, 135, 135, 135], [135, 135, 135, 135, 135, 135, 140, 167, 245, 362, 418, 349, 233, 163, 139, 135, 135, 135, 135, 135], [135, 135, 135, 135, 135, 136, 141, 171, 258, 390, 455, 377, 245, 165, 139, 135, 135, 135, 135, 135], [135, 135, 135, 135, 135, 136, 142, 172, 259, 387, 451, 376, 247, 166, 140, 135, 135, 135, 135, 135], [135, 135, 135, 135, 135, 135, 142, 170, 245, 357, 412, 348, 236, 163, 139, 135, 135, 135, 135, 135], [135, 135, 135, 135, 135, 135, 140, 163, 222, 308, 351, 303, 215, 158, 138, 135, 135, 135, 135, 135], [135, 135, 135, 135, 135, 135, 138, 154, 196, 256, 284, 252, 191, 152, 137, 135, 135, 135, 135, 135], [135, 135, 135, 135, 135, 135, 137, 147, 173, 209, 227, 207, 170, 145, 136, 135, 135, 135, 135, 135], [135, 135, 135, 135, 135, 135, 136, 142, 156, 175, 185, 174, 154, 140, 135, 135, 135, 135, 135, 135], [135, 135, 135, 135, 135, 135, 135, 138, 145, 154, 159, 154, 144, 137, 135, 135, 135, 135, 135, 135], [135, 135, 135, 135, 135, 135, 135, 136, 139, 143, 145, 143, 139, 136, 135, 135, 135, 135, 135, 135], [135, 135, 135, 135, 135, 135, 135, 135, 136, 138, 138, 138, 136, 135, 135, 135, 135, 135, 135, 135]]
  out "yx 4":u16[][](graph)=[[134, 132, 133, 133, 131, 134, 137, 129, 132, 138, 137, 132, 131, 134, 131, 132, 135, 133, 134, 132], [139, 137, 134, 132, 128, 131, 135, 137, 141, 132, 130, 136, 134, 127, 128, 135, 136, 133, 133, 136], [139, 135, 133, 129, 129, 132, 137, 140, 137, 136, 134, 134, 144, 144, 145, 137, 133, 133, 129, 132], [137, 135, 143, 138, 134, 130, 135, 141, 137, 129, 135, 136, 141, 140, 133, 128, 129, 127, 123, 126], [135, 138, 148, 151, 151, 144, 146, 141, 126, 119, 143, 148, 145, 135, 130, 127, 129, 126, 124, 130], [134, 134, 141, 146, 155, 147, 146, 144, 137, 132, 143, 161, 157, 137, 134, 135, 129, 127, 125, 129], [136, 138, 138, 134, 146, 143, 137, 140, 143, 140, 204, 249, 191, 141, 132, 137, 129, 126, 127, 126], [134, 137, 141, 140, 157, 153, 145, 137, 138, 220, 372, 326, 212, 151, 135, 134, 129, 130, 130, 122], [137, 138, 140, 135, 146, 158, 152, 153, 187, 287, 384, 308, 172, 144, 134, 134, 140, 131, 128, 126], [144, 145, 142, 131, 141, 149, 144, 189, 262, 389, 467, 337, 176, 139, 134, 138, 136, 130, 125, 135], [139, 141, 141, 136, 136, 141, 158, 235, 350, 389, 460, 371, 188, 136, 126, 137, 131, 130, 132, 139], [132, 136, 138, 134, 129, 152, 174, 238, 274, 350, 459, 372, 199, 139, 135, 137, 133, 132, 133, 133], [131, 135, 140, 142, 146, 166, 194, 211, 242, 298, 382, 363, 227, 143, 140, 137, 130, 131, 127, 131], [132, 131, 141, 143, 146, 164, 184, 208, 230, 257, 345, 384, 236, 154, 136, 137, 134, 135, 134, 128], [127, 125, 142, 142, 144, 160, 176, 188, 188, 229, 277, 273, 201, 146, 134, 132, 132, 131, 137, 127], [126, 126, 139, 145, 150, 153, 157, 165, 176, 191, 203, 223, 179, 146, 134, 126, 125, 130, 140, 134], [126, 128, 139, 143, 144, 149, 148, 150, 158, 181, 215, 216, 176, 147, 127, 123, 130, 133, 138, 138], [125, 129, 137, 137, 132, 144, 145, 142, 148, 165, 178, 180, 170, 140, 125, 128, 133, 131, 131, 131], [127, 135, 136, 136, 133, 145, 148, 147, 151, 152, 153, 156, 149, 131, 128, 130, 130, 129, 100, 57], [123, 131, 133, 132, 129, 136, 134, 132, 134, 127, 139, 156, 143, 129, 130, 127, 127, 96, 31, 0]]
  out "tilt 3":dbl=-2.58289224144748
  out "tilt 2":dbl=-0.0
  out "yx 3":dbl[][](graph)=[[134.9499399241804, 134.94993992735928, 134.94994011666108, 134.94994689756712, 134.9500925508678, 134.95195835824072, 134.96606856510073, 135.02781171692624, 135.17711556967282, 135.35038463951318, 135.37644338631844, 135.2244142667145, 135.0566683599304, 134.97501589369142, 134.95349979728468, 134.9502452829951, 134.94995575067753, 134.94994041978086, 134.94993993352654, 134.94993992425526], [134.9499399242392, 134.94993993335143, 134.94994048551243, 134.94996061318204, 134.9504006417102, 134.95613902239515, 135.00033887194684, 135.1975188179371, 135.6848005274849, 136.26787953279342, 136.37812751009096, 135.88507467377178, 135.31990636868235, 135.03838011568922, 134.96271419768144, 134.95105478828853, 134.94999871461098, 134.94994179737762, 134.94993996021208, 134.94993992456756], [134.9499399243755, 134.94993994751263, 134.94994137413596, 134.94999429541951, 134.95117181943053, 134.96680457262556, 135.08944178243138, 135.6471792762914, 137.05557441999412, 138.79216924098975, 139.1862015556717, 137.7720988416936, 136.08594260181818, 135.22623709815605, 134.99054428971715, 134.95354544667816, 134.95013337154785, 134.9499461954365, 134.94994004699086, 134.94993992560194], [134.9499399246508, 134.9499399766896, 134.94994324170767, 134.9500664949676, 134.95285767123644, 134.9905805974951, 135.29197712506408, 136.68928195160558, 140.2943015429152, 144.87209202520933, 146.0804514174922, 142.49432006079542, 138.03974585043812, 135.71454651806232, 135.06426567821296, 134.96026871083725, 134.95050376136743, 134.94995852176808, 134.94994029479477, 134.9499399286114], [134.94993992513238, 134.94994002880847, 134.9499466478417, 134.95020091934956, 134.95606140258818, 135.0366918898231, 135.69279059897846, 138.79340481913627, 146.9654860105327, 157.64667072832867, 160.85486247623967, 152.81483574912534, 142.39413724374913, 136.82421988875507, 135.23507473891496, 134.9761498161115, 134.95139564938893, 134.94998877732283, 134.9499409147641, 134.94993993628518], [134.94993992585512, 134.9499401088182, 134.94995199483336, 134.95041664734075, 134.96131619259967, 135.11397343522592, 136.3790462064828, 142.4730198216657, 158.8790208441416, 180.93910878077205, 188.35523286759542, 172.4224030399425, 150.83684784044036, 139.01967101628068, 135.5798684105343, 135.00885358099595, 134.9532691243449, 134.95005359864493, 134.94994226937763, 134.94993995338328], [134.94993992677044, 134.94994021278094, 134.9499591192651, 134.9507112446351, 134.9686673534806, 135.22467914697657, 137.38529540200508, 147.99371367830858, 177.1626612565863, 217.4933948282034, 232.47610173976352, 204.57391598322062, 164.98273190369258, 142.77759703368173, 136.18266740194838, 135.067240881991, 134.95668419865305, 134.95017422189753, 134.9499448422802, 134.94993998652603], [134.94993992771643, 134.94994032375197, 134.94996696276223, 134.95104537205142, 134.97724801441615, 135.35754874851784, 138.62610515879672, 154.9829250269071, 200.9121974656826, 266.1833916769077, 292.70844833509454, 249.53822746968171, 185.24054551190682, 148.28615834582135, 137.08680810677933, 135.15682157054144, 134.96204215389344, 134.9503676918799, 134.94994906001668, 134.9499400420418], [134.94993992844917, 134.9499404142072, 134.94997366164986, 134.95134330815011, 134.9852126741441, 135.48561484892466, 139.8653812079921, 162.2034789879957, 226.25240402236568, 319.76667293534297, 360.9972158488822, 302.00378062405514, 209.54547788534947, 155.07644810248232, 138.23106825076442, 135.27314427366477, 134.9691766154357, 134.95063172764435, 134.94995495675587, 134.94994012151983], [134.9499399287403, 134.94994045650395, 134.94997721276198, 134.9515180789105, 134.99029722741122, 135.57352237519683, 140.77184110307024, 167.7923464492414, 246.89484023274008, 365.50404198157094, 421.8565748548583, 350.67844211616676, 232.96067873012018, 161.85531161044693, 139.41269987928794, 135.39720733685098, 134.9770250080548, 134.95093096672227, 134.94996183471605, 134.94994021684226], [134.94993992849118, 134.94994043640807, 134.94997643100024, 134.95151194204726, 134.99084147582073, 135.5929551842416, 141.05798134930382, 170.0075144708553, 256.5296089893872, 389.71463620222283, 457.5145618765073, 381.72054110319846, 249.01937827205404, 166.8098382563467, 140.32667534700894, 135.49820697311725, 134.983720326872, 134.95119750726576, 134.9499682125082, 134.94994030863182], [134.9499399277865, 134.94994036077816, 134.94997158388938, 134.95132699999905, 134.9866590435521, 135.53727170643032, 140.6263523990655, 168.09841752653173, 251.91399794815555, 384.31779281506203, 456.188523741524, 384.9926156643361, 252.54789534583398, 168.36825911489854, 140.6880467984346, 135.54526182704842, 134.9872592928021, 134.95135348956995, 134.94997227582044, 134.9499403715282], [134.94993992684806, 134.9499402538122, 134.9499642447973, 134.95102404516157, 134.97913970274232, 135.4251444331188, 139.62277814467214, 162.7138185076788, 234.62321436824195, 351.1603067109318, 418.33274806566635, 359.3741389882056, 242.34024265108616, 165.99980001957445, 140.37436140417114, 135.5225334124144, 134.98646058106442, 134.95134736436037, 134.94997269747478, 134.94994038526414], [134.94993992592282, 134.9499401446257, 134.94995647337814, 134.950690492316, 134.9705083799166, 135.29051466181093, 138.35733406876116, 155.54824628152502, 210.18839196260438, 301.0031932604985, 356.38894633390987, 313.37672805424427, 221.8190134711307, 160.5045653869426, 139.49221100179582, 135.43777809191963, 134.98159750329054, 134.9511812300633, 134.94996933307283, 134.9499403451447], [134.94993992518144, 134.9499400547628, 134.94994989920195, 134.9504002203048, 134.96277382392358, 135.1661515967061, 137.15083241008162, 148.48679306481972, 185.257795483346, 247.91732907184903, 288.22432283313475, 260.6065268611577, 197.19431924159687, 153.57999849674306, 138.31914540355606, 135.3181027838093, 134.97424805969266, 134.95090968025312, 134.94996330027695, 134.94994026462038], [134.94993992468102, 134.94993999268974, 134.94994524998094, 134.95018996984396, 134.957033258436, 135.07152511186666, 136.20918456216842, 142.83016730799508, 164.74653139327864, 203.02587605732356, 228.92656753752044, 213.33716461279698, 174.45656392892576, 146.98071889707984, 137.1636297824914, 135.19605544413935, 134.9664732576074, 134.95061101458074, 134.94995638305036, 134.94994016805256], [134.94993992439154, 134.9499399560085, 134.94994244295364, 134.95006024371096, 134.95341270228673, 135.0105042699609, 135.58813907275237, 139.01338701012077, 150.58257519548158, 171.2886059332258, 185.9892697964509, 178.2651220948289, 157.16126791004353, 141.8318358970998, 136.2383107445387, 135.09567794087377, 134.9599009491106, 134.9503512958373, 134.9499501892666, 134.94994007892015], [134.94993992424656, 134.94993993726652, 134.94994097935242, 134.94999120886175, 134.95144597098445, 134.97666310920044, 135.2364481915343, 136.8059712244634, 142.21488996082928, 152.13215560075128, 159.50408959311955, 156.15159816719995, 146.01143827606762, 138.43698279352918, 135.6141413637186, 135.02638359552378, 134.95525589339, 134.95016329298372, 134.94994559517744, 134.94994001114426], [134.94993992418335, 134.94993992893268, 134.9499403157216, 134.9499592872286, 134.95051846595143, 134.9603845824188, 135.06387381369134, 135.7008895595083, 137.94060580442965, 142.14648714791187, 145.4135045626645, 144.14245480887547, 139.82958484153738, 136.51503706220902, 135.25325470367568, 134.98545764144671, 134.9524529428354, 134.95004735909862, 134.9499426993504, 134.94993996746348], [134.94993992415925, 134.94993992569383, 134.9499400528618, 134.9499463999834, 134.95013678793697, 134.953555979578, 134.99007309897698, 135.21907552736644, 136.04047085432785, 137.6198954094083, 138.89968668772067, 138.48041932174903, 136.8567055293293, 135.57218309032115, 135.07263359499544, 134.9645577701783, 134.95099223440712, 134.94998569652057, 134.94994112713866, 134.94993994325185]]
  out "yx 2":u16[][](graph)=[[131, 129, 135, 132, 132, 139, 137, 122, 139, 139, 137, 129, 133, 135, 129, 136, 135, 133, 135, 131], [138, 136, 137, 132, 126, 133, 136, 137, 144, 125, 134, 139, 132, 123, 130, 141, 134, 133, 133, 145], [141, 137, 127, 128, 130, 136, 140, 141, 136, 137, 134, 135, 152, 146, 152, 130, 134, 134, 123, 128], [138, 128, 144, 130, 130, 126, 137, 144, 136, 127, 139, 136, 143, 138, 126, 125, 130, 122, 121, 130], [137, 144, 153, 150, 148, 141, 148, 139, 121, 118, 152, 148, 145, 131, 131, 128, 131, 127, 126, 134], [133, 132, 146, 154, 161, 146, 149, 144, 136, 131, 147, 167, 157, 133, 136, 139, 126, 127, 125, 129], [137, 138, 137, 130, 145, 140, 136, 142, 144, 138, 219, 263, 181, 134, 131, 138, 129, 125, 130, 125], [136, 139, 143, 142, 163, 151, 143, 135, 136, 232, 399, 322, 200, 147, 135, 134, 129, 134, 131, 119], [132, 135, 140, 138, 149, 161, 154, 150, 186, 294, 392, 300, 157, 142, 134, 135, 146, 129, 126, 132], [145, 146, 141, 129, 142, 152, 142, 186, 259, 394, 472, 336, 174, 138, 134, 140, 133, 130, 124, 140], [144, 144, 144, 138, 140, 139, 155, 233, 355, 389, 462, 378, 192, 136, 124, 137, 131, 130, 138, 139], [134, 136, 138, 132, 123, 148, 167, 240, 272, 344, 465, 384, 205, 140, 138, 138, 135, 134, 131, 129], [129, 136, 140, 142, 144, 163, 195, 208, 238, 289, 380, 379, 240, 145, 141, 138, 129, 131, 125, 133], [135, 134, 140, 144, 145, 163, 181, 206, 230, 244, 332, 409, 251, 160, 135, 138, 137, 138, 142, 125], [131, 122, 144, 143, 138, 158, 176, 193, 182, 218, 275, 277, 209, 147, 135, 131, 131, 124, 139, 129], [126, 121, 137, 144, 150, 153, 157, 165, 173, 192, 191, 231, 186, 150, 137, 126, 123, 129, 144, 139], [130, 127, 139, 145, 148, 151, 149, 150, 155, 169, 212, 228, 185, 155, 128, 119, 133, 133, 135, 138], [123, 119, 136, 143, 127, 142, 146, 142, 143, 160, 177, 175, 180, 147, 124, 128, 134, 131, 128, 127], [126, 140, 134, 143, 130, 143, 154, 146, 153, 152, 152, 153, 156, 131, 128, 131, 129, 130, 129, 0], [117, 131, 131, 137, 126, 134, 139, 129, 138, 130, 124, 158, 154, 128, 133, 128, 123, 132, 0, 0]]
  out "Numeric":i32=38
  out "#function calls":i32=18
  out "residue":dbl=513.1920909975838
  in  "anal method":T3(ring)
  in  "tilt":dbl=20.0 format="%#_13g"
  in  "indexing variable":i32
  out "Z":i32=16
  out "FWHMz":T4(graph)={"X Values"=[0.49091547409651104, 0.5436936843186253, 0.5964718945407396, 0.6492501047628538, 0.7020283149849681, 0.7548065252070824, 0.8075847354291966, 0.8603629456513109, 0.9131411558734251, 0.9659193660955394, 1.0186975763176538, 1.0714757865397682, 1.1242539967618825, 1.177032206983997, 1.2298104172061113, 1.2825886274282257, 1.33536683765034, 1.3881450478724544, 1.4409232580945688, 1.4937014683166832, 1.5464796785387975, 1.599257888760912, 1.6520360989830263, 1.7048143092051407, 1.757592519427255, 1.8103707296493694, 1.8631489398714838, 1.9159271500935982, 1.9687053603157125, 2.0214835705378267, 2.074261780759941, 2.1270399909820554, 2.17981820120417, 2.232596411426284, 2.2853746216483986, 2.338152831870513, 2.3909310420926273, 2.4437092523147417, 2.496487462536856, 2.5492656727589704, 2.602043882981085, 2.654822093203199, 2.7076003034253135, 2.760378513647428, 2.8131567238695423, 2.8659349340916567, 2.918713144313771, 2.9714913545358854, 3.024269564758, 3.077047774980114], "Histogram: h(x)"=[1, 0, 1, 1, 0, 0, 1, 0, 0, 1, 0, 2, 1, 0, 0, 1, 2, 0, 0, 2, 1, 0, 0, 2, 8, 1, 1, 2, 1, 1, 1, 2, 2, 0, 0, 0, 0, 0, 0, 0, 1, 0, 0, 0, 0, 0, 2, 0, 0, 1]}
  out "FWHMy":T4(graph)={"X Values"=[0.38574742692294495, 0.39994402150286423, 0.4141406160827835, 0.4283372106627028, 0.4425338052426221, 0.4567303998225414, 0.47092699440246066, 0.48512358898237995, 0.49932018356229924, 0.5135167781422185, 0.5277133727221378, 0.5419099673020571, 0.5561065618819764, 0.5703031564618957, 0.584499751041815, 0.5986963456217342, 0.6128929402016535, 0.6270895347815728, 0.6412861293614921, 0.6554827239414114, 0.6696793185213307, 0.68387591310125, 0.6980725076811692, 0.7122691022610885, 0.7264656968410078, 0.7406622914209271, 0.7548588860008464, 0.7690554805807657, 0.783252075160685, 0.7974486697406042, 0.8116452643205235, 0.8258418589004428, 0.8400384534803621, 0.8542350480602814, 0.8684316426402007, 0.88262823722012, 0.8968248318000392, 0.9110214263799585, 0.9252180209598778, 0.9394146155397971, 0.9536112101197164, 0.9678078046996357, 0.982004399279555, 0.9962009938594742, 1.0103975884393934, 1.0245941830193126, 1.0387907775992318, 1.052987372179151, 1.0671839667590701, 1.0813805613389893], "Histogram: h(x)"=[2, 2, 3, 8, 1, 5, 5, 2, 3, 1, 1, 0, 0, 1, 1, 0, 2, 0, 0, 0, 0, 0, 0, 0, 0, 0, 0, 0, 1, 0, 0, 0, 0, 0, 0, 0, 0, 0, 0, 0, 0, 0, 0, 0, 0, 0, 0, 0, 0, 1]}
  out "FWHMx":T4(graph)={"X Values"=[0.038327908101687, 0.114983724305061, 0.191639540508435, 0.26829535671180904, 0.34495117291518307, 0.4216069891185571, 0.4982628053219311, 0.5749186215253052, 0.6515744377286792, 0.7282302539320532, 0.8048860701354272, 0.8815418863388013, 0.9581977025421753, 1.0348535187455492, 1.1115093349489231, 1.188165151152297, 1.264820967355671, 1.3414767835590449, 1.4181325997624188, 1.4947884159657927, 1.5714442321691666, 1.6481000483725405, 1.7247558645759145, 1.8014116807792884, 1.8780674969826623, 1.9547233131860362, 2.03137912938941, 2.108034945592784, 2.184690761796158, 2.261346577999532, 2.338002394202906, 2.4146582104062797, 2.4913140266096536, 2.5679698428130275, 2.6446256590164015, 2.7212814752197754, 2.7979372914231493, 2.874593107626523, 2.951248923829897, 3.027904740033271, 3.104560556236645, 3.181216372440019, 3.257872188643393, 3.3345280048467667, 3.4111838210501406, 3.4878396372535145, 3.5644954534568885, 3.6411512696602624, 3.7178070858636363, 3.79446290206701], "Histogram: h(x)"=[1, 0, 0, 0, 0, 0, 0, 0, 2, 3, 4, 8, 6, 4, 1, 2, 1, 1, 0, 2, 0, 0, 1, 0, 0, 0, 0, 1, 0, 0, 0, 0, 0, 0, 0, 0, 0, 0, 0, 0, 0, 0, 0, 0, 0, 0, 0, 1, 0, 1]}
  in  "intervals":i32=50
  out "FWHMz [um]":dbl=1.894751855635071
  out "xz MIP":i32[][](graph)
  out "zy":u16[][](graph)=[[116, 118, 110, 138, 128, 114, 112, 101, 106, 102, 107, 97, 98, 94, 107, 101, 98, 95, 103, 100, 103, 98, 96, 96, 99, 96, 99, 104, 92, 91, 95, 97, 94, 108, 87, 102, 95, 93, 95, 94], [119, 124, 132, 144, 140, 124, 120, 113, 117, 110, 114, 102, 108, 103, 106, 104, 107, 102, 101, 100, 109, 106, 101, 103, 99, 100, 104, 107, 97, 97, 105, 103, 96, 105, 93, 105, 103, 100, 98, 98], [122, 130, 146, 154, 142, 131, 129, 121, 118, 110, 116, 106, 109, 107, 106, 102, 110, 102, 99, 98, 107, 106, 102, 103, 101, 104, 101, 105, 99, 101, 107, 99, 98, 103, 96, 101, 102, 100, 98, 100], [126, 135, 156, 168, 146, 146, 139, 124, 120, 111, 114, 108, 104, 109, 106, 97, 103, 102, 104, 104, 108, 105, 103, 99, 102, 104, 102, 105, 99, 102, 103, 98, 100, 107, 99, 103, 104, 102, 100, 100], [130, 137, 156, 178, 160, 155, 138, 122, 122, 113, 108, 103, 101, 105, 104, 91, 98, 107, 108, 112, 108, 107, 106, 99, 104, 102, 105, 107, 106, 102, 98, 105, 102, 109, 105, 105, 105, 101, 101, 98], [131, 146, 174, 188, 173, 160, 151, 134, 127, 122, 110, 110, 113, 109, 111, 99, 104, 105, 104, 109, 104, 105, 102, 104, 105, 103, 105, 107, 109, 108, 105, 109, 104, 103, 106, 104, 97, 102, 105, 100], [127, 144, 191, 195, 195, 171, 155, 140, 132, 125, 115, 116, 112, 105, 111, 104, 106, 108, 104, 108, 110, 108, 104, 105, 109, 103, 103, 106, 108, 108, 109, 109, 105, 102, 103, 100, 96, 106, 105, 102], [130, 148, 199, 220, 211, 185, 170, 150, 135, 125, 119, 118, 107, 104, 104, 102, 106, 115, 111, 111, 115, 115, 111, 101, 112, 103, 99, 106, 110, 110, 111, 114, 107, 104, 102, 104, 103, 102, 102, 98], [136, 162, 218, 248, 238, 216, 183, 159, 142, 129, 120, 114, 107, 106, 106, 103, 104, 112, 111, 111, 117, 115, 112, 97, 110, 103, 102, 102, 107, 109, 110, 115, 111, 107, 105, 109, 105, 102, 102, 98], [142, 171, 233, 264, 271, 245, 194, 163, 144, 132, 120, 111, 108, 107, 110, 107, 107, 111, 110, 111, 117, 114, 113, 99, 104, 105, 103, 101, 106, 109, 111, 117, 114, 109, 107, 111, 108, 104, 101, 102], [151, 178, 232, 275, 306, 283, 208, 160, 139, 134, 120, 108, 109, 110, 112, 109, 112, 115, 112, 115, 115, 115, 113, 105, 103, 105, 104, 102, 107, 109, 113, 114, 114, 110, 110, 108, 108, 105, 104, 107], [169, 195, 242, 290, 339, 323, 226, 151, 134, 126, 118, 107, 113, 113, 113, 109, 120, 120, 116, 116, 118, 119, 111, 110, 107, 105, 107, 105, 107, 110, 112, 114, 115, 109, 113, 105, 106, 106, 111, 113], [179, 214, 258, 316, 385, 374, 243, 146, 132, 113, 112, 102, 112, 108, 113, 103, 115, 117, 129, 125, 122, 125, 110, 107, 110, 106, 111, 105, 102, 113, 114, 122, 123, 111, 113, 101, 113, 103, 112, 109], [196, 240, 271, 349, 469, 437, 250, 147, 124, 110, 108, 106, 106, 103, 108, 99, 108, 117, 131, 133, 118, 121, 104, 105, 112, 106, 110, 105, 108, 117, 122, 128, 130, 116, 109, 103, 121, 104, 110, 105], [232, 266, 287, 387, 554, 509, 252, 141, 117, 115, 107, 116, 111, 105, 107, 102, 111, 129, 117, 129, 110, 118, 100, 102, 116, 109, 105, 107, 113, 117, 132, 133, 127, 116, 117, 113, 118, 104, 115, 115], [240, 272, 314, 422, 623, 567, 255, 137, 130, 114, 104, 115, 112, 106, 111, 106, 113, 125, 126, 136, 123, 123, 106, 109, 116, 118, 109, 111, 114, 126, 141, 146, 129, 112, 118, 112, 120, 109, 122, 126], [252, 259, 318, 458, 696, 578, 273, 147, 143, 114, 115, 112, 112, 105, 114, 111, 117, 123, 132, 139, 128, 124, 112, 109, 117, 114, 114, 115, 112, 132, 154, 152, 143, 118, 123, 112, 120, 115, 124, 121], [246, 257, 310, 461, 678, 563, 299, 170, 143, 118, 111, 108, 113, 110, 115, 118, 120, 128, 141, 141, 130, 120, 122, 111, 120, 120, 116, 113, 117, 131, 165, 158, 150, 125, 129, 121, 121, 119, 130, 124], [223, 252, 305, 421, 600, 551, 315, 187, 143, 119, 114, 114, 115, 113, 117, 116, 121, 127, 146, 148, 132, 124, 119, 113, 118, 122, 115, 113, 116, 133, 174, 175, 152, 128, 130, 128, 124, 118, 125, 123], [202, 231, 291, 394, 555, 542, 325, 208, 148, 120, 115, 115, 114, 111, 117, 114, 115, 129, 145, 151, 145, 131, 123, 116, 112, 118, 116, 118, 110, 136, 187, 188, 155, 129, 135, 130, 125, 121, 126, 119], [191, 210, 251, 347, 490, 497, 314, 231, 156, 128, 117, 113, 114, 110, 120, 118, 110, 128, 139, 147, 150, 135, 120, 120, 108, 114, 116, 118, 104, 138, 199, 197, 156, 133, 135, 130, 126, 123, 130, 114], [182, 191, 208, 297, 417, 432, 287, 229, 161, 134, 130, 118, 116, 112, 116, 127, 115, 127, 135, 144, 153, 145, 114, 108, 111, 119, 114, 117, 107, 141, 198, 222, 167, 142, 142, 135, 128, 125, 130, 113], [164, 171, 185, 254, 355, 352, 258, 214, 172, 137, 127, 121, 114, 113, 111, 114, 130, 139, 141, 158, 156, 140, 119, 114, 112, 120, 120, 118, 113, 157, 236, 253, 178, 148, 154, 148, 130, 134, 132, 126], [154, 160, 169, 222, 282, 295, 228, 179, 175, 147, 128, 120, 113, 114, 113, 110, 134, 147, 146, 170, 159, 147, 118, 117, 111, 113, 121, 114, 120, 177, 266, 273, 184, 160, 157, 152, 137, 140, 128, 127], [151, 147, 164, 201, 236, 234, 196, 171, 163, 149, 131, 117, 117, 116, 115, 120, 139, 151, 146, 166, 157, 156, 115, 115, 107, 110, 114, 114, 130, 194, 289, 284, 196, 172, 154, 157, 154, 147, 132, 120], [152, 144, 156, 182, 205, 193, 180, 170, 161, 149, 136, 123, 120, 119, 119, 127, 146, 147, 147, 162, 168, 164, 116, 111, 107, 111, 119, 118, 145, 217, 310, 281, 199, 181, 152, 157, 164, 147, 137, 121], [150, 147, 148, 168, 179, 164, 162, 160, 157, 150, 138, 123, 120, 121, 121, 128, 146, 141, 149, 160, 177, 165, 123, 112, 112, 114, 122, 121, 165, 247, 324, 277, 217, 197, 163, 161, 163, 150, 141, 124], [151, 145, 144, 156, 163, 150, 150, 150, 147, 145, 135, 123, 123, 124, 124, 133, 146, 142, 149, 170, 190, 164, 128, 118, 117, 118, 124, 129, 196, 273, 329, 282, 253, 213, 180, 171, 165, 152, 143, 125], [169, 159, 144, 132, 156, 149, 140, 140, 144, 137, 138, 133, 130, 134, 134, 150, 153, 146, 146, 181, 204, 161, 126, 119, 117, 117, 122, 145, 221, 291, 350, 294, 272, 215, 197, 191, 171, 154, 148, 129], [180, 175, 142, 139, 156, 143, 132, 134, 142, 145, 158, 143, 143, 139, 136, 145, 158, 152, 146, 192, 213, 164, 130, 117, 119, 117, 131, 168, 232, 303, 344, 310, 273, 233, 198, 185, 164, 158, 149, 134], [193, 171, 143, 145, 161, 143, 131, 132, 146, 148, 161, 148, 136, 143, 136, 141, 161, 152, 154, 204, 224, 167, 129, 114, 115, 126, 132, 192, 250, 335, 342, 336, 291, 233, 208, 179, 182, 168, 149, 127], [192, 167, 149, 142, 152, 147, 128, 136, 147, 160, 157, 143, 137, 154, 153, 147, 159, 159, 176, 196, 231, 167, 138, 124, 128, 131, 138, 178, 230, 298, 274, 313, 288, 239, 203, 194, 205, 172, 149, 128], [200, 160, 147, 144, 143, 144, 128, 144, 148, 156, 150, 148, 148, 159, 164, 156, 155, 165, 198, 209, 234, 165, 146, 128, 133, 128, 144, 170, 209, 250, 234, 274, 256, 241, 215, 213, 196, 165, 153, 127], [216, 153, 142, 142, 140, 134, 128, 142, 144, 142, 152, 146, 152, 162, 164, 158, 154, 178, 213, 232, 228, 172, 152, 133, 136, 130, 146, 165, 192, 203, 216, 241, 236, 236, 227, 225, 193, 161, 154, 124], [231, 150, 136, 140, 138, 127, 125, 133, 136, 132, 148, 136, 150, 158, 157, 155, 156, 199, 215, 238, 216, 180, 151, 135, 136, 128, 148, 151, 174, 172, 190, 210, 221, 215, 220, 224, 209, 159, 146, 122], [224, 148, 125, 132, 135, 127, 123, 127, 132, 129, 132, 124, 137, 142, 140, 143, 153, 193, 203, 205, 198, 172, 143, 134, 128, 129, 143, 139, 156, 154, 157, 182, 197, 186, 193, 217, 211, 154, 139, 124], [199, 145, 121, 128, 124, 112, 111, 113, 122, 119, 120, 119, 123, 124, 124, 130, 135, 172, 168, 175, 177, 155, 132, 126, 121, 129, 134, 129, 132, 140, 139, 159, 163, 171, 186, 224, 202, 152, 128, 116], [158, 131, 116, 119, 113, 106, 107, 106, 113, 111, 113, 114, 110, 115, 118, 121, 121, 146, 133, 150, 153, 137, 122, 118, 117, 127, 126, 124, 117, 129, 131, 139, 144, 158, 174, 208, 168, 134, 114, 109], [131, 116, 112, 114, 110, 107, 107, 108, 111, 111, 114, 117, 109, 108, 113, 116, 109, 123, 125, 133, 133, 125, 117, 114, 114, 114, 118, 122, 117, 123, 125, 126, 132, 135, 158, 172, 143, 115, 105, 105], [104, 95, 98, 98, 94, 90, 91, 94, 97, 98, 98, 102, 101, 96, 99, 99, 94, 102, 108, 110, 111, 105, 102, 99, 99, 100, 98, 100, 102, 104, 104, 104, 105, 107, 117, 123, 104, 90, 92, 94]]
  out "zx":u16[][](graph)=[[0, 0, 114, 104, 112, 118, 122, 117, 103, 97, 108, 117, 114, 121, 126, 126, 124, 124, 135, 135, 128, 120, 125, 123, 114, 112, 117, 110, 103, 106, 108, 105, 104, 106, 99, 95, 94, 109, 109, 110], [0, 145, 129, 118, 118, 119, 121, 116, 110, 104, 107, 111, 114, 121, 126, 127, 124, 138, 152, 156, 140, 130, 131, 134, 121, 116, 118, 121, 116, 110, 111, 110, 107, 107, 105, 102, 104, 109, 108, 109], [146, 146, 138, 129, 125, 122, 117, 114, 115, 116, 109, 109, 112, 121, 127, 129, 135, 157, 172, 152, 142, 137, 141, 141, 128, 122, 129, 128, 122, 115, 113, 113, 109, 114, 112, 108, 107, 110, 109, 110], [143, 147, 145, 137, 127, 118, 112, 106, 114, 114, 112, 112, 115, 120, 128, 132, 146, 175, 169, 154, 146, 148, 153, 149, 134, 133, 134, 127, 117, 114, 110, 113, 114, 116, 115, 111, 109, 110, 111, 112], [159, 154, 152, 141, 120, 111, 105, 111, 112, 112, 112, 115, 117, 120, 130, 135, 150, 167, 169, 160, 160, 153, 156, 147, 141, 137, 135, 122, 115, 112, 107, 111, 116, 117, 115, 113, 111, 111, 115, 119], [183, 164, 156, 143, 127, 110, 114, 116, 116, 114, 113, 112, 110, 123, 132, 133, 144, 162, 174, 180, 173, 164, 162, 159, 150, 142, 136, 123, 119, 113, 113, 116, 119, 120, 117, 116, 117, 112, 114, 120], [203, 172, 157, 148, 139, 120, 118, 118, 118, 115, 115, 112, 112, 118, 132, 140, 151, 166, 182, 190, 195, 182, 177, 173, 162, 149, 134, 125, 129, 119, 116, 119, 121, 123, 118, 119, 115, 111, 114, 119], [216, 175, 157, 147, 126, 120, 120, 121, 119, 116, 115, 115, 119, 130, 137, 152, 166, 183, 182, 200, 211, 195, 188, 182, 175, 163, 144, 130, 129, 124, 123, 122, 125, 127, 121, 113, 111, 109, 114, 119], [240, 179, 155, 143, 129, 125, 125, 123, 121, 115, 116, 115, 123, 138, 149, 163, 181, 202, 219, 240, 238, 219, 198, 189, 183, 174, 148, 139, 132, 131, 132, 129, 129, 134, 120, 113, 112, 112, 117, 121], [248, 179, 162, 144, 130, 128, 127, 123, 117, 114, 114, 112, 117, 128, 139, 152, 187, 226, 257, 279, 271, 246, 218, 194, 194, 191, 165, 154, 144, 137, 137, 133, 133, 128, 120, 118, 117, 115, 120, 124], [214, 188, 166, 143, 127, 124, 124, 120, 116, 114, 117, 116, 118, 124, 126, 157, 210, 272, 304, 318, 306, 270, 232, 208, 217, 202, 180, 164, 150, 140, 137, 135, 128, 120, 121, 123, 119, 114, 116, 120], [248, 195, 172, 145, 125, 121, 120, 121, 118, 116, 115, 117, 118, 123, 130, 165, 232, 297, 347, 360, 339, 295, 263, 248, 231, 207, 184, 165, 148, 139, 136, 134, 129, 119, 124, 129, 124, 118, 121, 126], [278, 216, 176, 150, 134, 131, 131, 126, 117, 119, 114, 113, 109, 114, 134, 177, 232, 316, 385, 409, 385, 343, 316, 291, 257, 218, 182, 164, 148, 142, 138, 132, 123, 123, 131, 137, 129, 127, 130, 132], [282, 215, 168, 151, 142, 139, 144, 138, 132, 124, 115, 111, 110, 114, 140, 176, 242, 338, 431, 475, 469, 424, 362, 307, 268, 221, 188, 170, 158, 151, 140, 131, 126, 129, 138, 142, 135, 135, 138, 139], [267, 208, 164, 148, 149, 144, 150, 154, 149, 136, 117, 114, 114, 121, 133, 175, 247, 355, 458, 535, 554, 495, 416, 341, 273, 229, 195, 175, 162, 154, 145, 136, 130, 132, 134, 138, 137, 144, 147, 147], [249, 216, 172, 165, 159, 150, 161, 166, 164, 145, 118, 108, 113, 117, 131, 165, 241, 344, 480, 623, 623, 560, 482, 388, 307, 252, 210, 179, 156, 144, 139, 132, 126, 124, 133, 138, 142, 154, 157, 152], [233, 218, 187, 179, 170, 163, 163, 169, 167, 154, 128, 117, 113, 116, 128, 160, 219, 322, 478, 647, 696, 630, 535, 414, 336, 284, 227, 189, 163, 146, 134, 127, 120, 125, 138, 144, 150, 160, 162, 154], [209, 206, 191, 194, 185, 175, 169, 165, 172, 164, 144, 127, 119, 119, 126, 152, 200, 279, 436, 590, 678, 655, 557, 443, 366, 291, 231, 189, 168, 152, 138, 126, 123, 130, 147, 148, 151, 159, 155, 164], [177, 190, 181, 185, 190, 183, 176, 176, 185, 179, 161, 134, 121, 119, 122, 133, 170, 265, 382, 511, 600, 629, 571, 473, 387, 296, 231, 189, 167, 156, 140, 129, 126, 137, 144, 143, 144, 152, 171, 173], [159, 176, 172, 174, 184, 191, 185, 180, 185, 193, 170, 138, 114, 111, 116, 123, 158, 234, 331, 442, 555, 607, 577, 512, 407, 303, 233, 189, 166, 156, 142, 133, 131, 138, 139, 137, 144, 164, 184, 177], [147, 164, 167, 166, 179, 200, 198, 177, 181, 188, 176, 138, 118, 113, 123, 124, 144, 186, 266, 371, 490, 576, 571, 524, 408, 310, 245, 193, 174, 156, 142, 140, 136, 135, 136, 136, 146, 169, 191, 185], [134, 147, 155, 157, 161, 190, 189, 172, 170, 178, 168, 140, 120, 118, 116, 119, 134, 161, 217, 311, 417, 505, 526, 490, 420, 339, 267, 201, 177, 155, 141, 138, 139, 136, 135, 134, 146, 173, 183, 185], [127, 133, 142, 145, 153, 180, 182, 167, 159, 167, 160, 134, 111, 113, 113, 119, 132, 153, 196, 269, 355, 446, 491, 468, 424, 359, 257, 199, 170, 149, 141, 140, 142, 142, 138, 137, 145, 160, 172, 179], [123, 123, 133, 137, 145, 162, 171, 159, 153, 161, 157, 130, 122, 115, 115, 123, 134, 147, 181, 214, 282, 382, 430, 435, 413, 351, 270, 194, 157, 143, 135, 137, 140, 141, 134, 128, 139, 153, 169, 194], [115, 120, 125, 125, 134, 144, 150, 148, 144, 149, 140, 145, 132, 118, 117, 124, 132, 145, 156, 183, 236, 307, 355, 372, 378, 357, 293, 218, 163, 148, 140, 131, 130, 131, 128, 127, 136, 148, 174, 201], [117, 119, 118, 122, 128, 133, 139, 146, 140, 142, 151, 151, 137, 118, 118, 124, 127, 133, 147, 169, 205, 245, 285, 318, 360, 368, 322, 245, 182, 158, 146, 131, 121, 125, 126, 125, 134, 140, 168, 193], [120, 123, 123, 121, 126, 133, 150, 153, 146, 145, 150, 147, 133, 119, 120, 125, 120, 130, 146, 160, 179, 204, 231, 283, 324, 328, 317, 249, 188, 165, 146, 132, 128, 124, 124, 122, 125, 143, 166, 176], [120, 127, 126, 122, 123, 130, 141, 138, 136, 135, 140, 135, 128, 121, 124, 121, 122, 139, 148, 154, 163, 178, 203, 246, 275, 278, 271, 232, 183, 171, 153, 137, 130, 125, 125, 123, 135, 146, 154, 169], [122, 127, 125, 120, 119, 119, 120, 132, 134, 133, 135, 131, 128, 127, 120, 121, 124, 137, 145, 148, 156, 158, 176, 214, 240, 248, 247, 218, 200, 179, 147, 137, 130, 125, 129, 138, 147, 145, 151, 166], [126, 126, 122, 121, 123, 128, 120, 127, 132, 133, 134, 128, 129, 127, 120, 119, 123, 132, 140, 152, 156, 154, 162, 183, 206, 217, 230, 222, 210, 173, 145, 138, 135, 131, 136, 144, 140, 146, 152, 164], [128, 126, 121, 122, 125, 125, 122, 123, 127, 133, 134, 120, 119, 124, 118, 118, 124, 133, 148, 157, 161, 152, 149, 159, 178, 192, 196, 207, 201, 177, 144, 141, 138, 135, 141, 151, 145, 142, 146, 153], [128, 119, 117, 119, 121, 127, 129, 128, 128, 134, 138, 124, 120, 124, 124, 124, 129, 142, 149, 153, 152, 147, 139, 144, 162, 169, 174, 187, 199, 183, 157, 144, 144, 142, 151, 155, 148, 143, 140, 153], [128, 120, 122, 124, 126, 135, 136, 129, 127, 133, 134, 129, 126, 129, 129, 129, 132, 137, 143, 141, 143, 143, 135, 139, 143, 152, 165, 174, 182, 184, 161, 151, 148, 143, 149, 152, 148, 146, 144, 154], [131, 129, 134, 132, 131, 136, 130, 127, 133, 132, 136, 135, 134, 133, 132, 130, 126, 133, 141, 143, 140, 140, 130, 123, 128, 144, 156, 161, 167, 170, 160, 153, 149, 154, 157, 160, 164, 158, 149, 146], [124, 137, 140, 134, 125, 123, 122, 129, 135, 132, 135, 140, 139, 137, 140, 127, 121, 129, 134, 138, 138, 132, 127, 124, 120, 133, 142, 151, 156, 158, 153, 148, 159, 167, 168, 166, 172, 173, 160, 0], [130, 126, 131, 123, 116, 116, 123, 125, 135, 129, 133, 141, 137, 132, 133, 129, 123, 119, 122, 130, 135, 123, 121, 121, 119, 123, 130, 140, 147, 146, 140, 147, 165, 175, 170, 167, 173, 175, 0, 0], [127, 121, 114, 115, 111, 118, 115, 119, 128, 126, 132, 141, 136, 131, 131, 129, 124, 114, 113, 129, 124, 114, 111, 116, 113, 114, 123, 134, 137, 129, 129, 139, 156, 170, 172, 172, 169, 0, 0, 0], [119, 113, 111, 114, 109, 116, 120, 123, 126, 122, 127, 137, 135, 129, 127, 124, 118, 108, 111, 114, 113, 108, 109, 112, 108, 109, 120, 129, 124, 125, 126, 131, 146, 158, 172, 174, 0, 0, 0, 0], [113, 111, 110, 111, 110, 114, 117, 120, 118, 115, 123, 126, 126, 121, 120, 120, 115, 110, 105, 108, 110, 104, 107, 111, 110, 111, 118, 117, 122, 125, 128, 132, 141, 150, 159, 0, 0, 0, 0, 0], [109, 112, 109, 86, 91, 102, 100, 106, 110, 113, 110, 97, 111, 105, 113, 120, 114, 110, 106, 108, 94, 95, 103, 110, 111, 110, 108, 94, 107, 124, 121, 132, 142, 144, 0, 0, 0, 0, 0, 0]]
  out "z2":dbl[][](graph)=[[159.0701335098287, 159.41572827638566, 160.23612601610066, 162.05277131711512, 165.80205397080528, 173.00664136653782, 185.87947907628242, 207.22866266650232, 240.01529312864716, 286.4851438838343, 346.97468715461525, 418.74214583875505, 495.3696866526853, 567.2603811213316, 623.4203914576874, 654.1570098456504, 653.8047551853026, 622.4299117092417, 565.8101756278546, 493.6979788264614, 417.0834176044964, 345.5082501781553, 285.3101931465353, 239.15382195262825, 206.6471767543749, 185.51669162287595, 172.79684694649484, 165.68937417471867, 161.99647637185342, 160.20993381896335], [140.0, 142.0, 146.0, 160.0, 173.0, 195.0, 211.0, 238.0, 271.0, 306.0, 339.0, 385.0, 469.0, 554.0, 623.0, 696.0, 678.0, 600.0, 555.0, 490.0, 417.0, 355.0, 282.0, 236.0, 205.0, 179.0, 163.0, 156.0, 156.0, 161.0]]
  in  "parameter bounds 2":T5={"amp min"=105.0, "amp max"=70000.0, "center min"=0.0, "center max"=100.0, "deviation min"=0.0, "deviation max"=10.0, "offset min"=50.0, "offset max"=200.0}
  in  "FWHM [um]":dbl[](array[numeric])=[2.0, 1.0, 0.8] format="%#_13g"
  in  "Nx2":i32=500
  in  "bg black/white":bool=TRUE
  out "X":dbl=56.0
  out "Y":dbl=4.0
  out "min":dbl
  out "max":dbl=3.8327908101687
  in  "color 3":T6={"color array"=[0, 16711680, 16776281, 16448250, 16776960, 16711680, 16448250, 16448250], "num of colors"=4, "max"=900.5, "min"=0.0} {"min" step=0.01 format="%_2f"; "max" step=0.1 format="%_3f"}
  in  "color 2":T6={"color array"=[0, 16711680, 16776281, 16448250, 16776960, 16711680, 16448250, 16448250], "num of colors"=4, "max"=699.6999999999998, "min"=100.0} {"min" step=0.01 format="%_2f"; "max" step=0.1 format="%_3f"}
  out "yx":u16[][](graph)=[[143, 145, 135, 125, 128, 126, 116, 109, 115, 118, 115, 115, 120, 126, 132, 134, 139, 166, 218, 266, 252, 193, 149, 130, 138, 142, 131, 134, 134, 135, 138, 136, 135, 126, 127, 128, 129, 127, 120, 112], [184, 178, 142, 119, 115, 114, 111, 111, 111, 105, 103, 105, 111, 120, 140, 157, 168, 202, 239, 257, 259, 231, 195, 175, 164, 146, 129, 131, 133, 127, 132, 139, 138, 130, 130, 135, 133, 122, 109, 108], [225, 211, 160, 126, 114, 116, 117, 114, 109, 112, 117, 116, 116, 123, 139, 168, 212, 252, 269, 291, 318, 344, 352, 315, 261, 205, 160, 151, 139, 129, 131, 134, 135, 130, 130, 136, 138, 135, 130, 126], [251, 215, 174, 150, 137, 132, 129, 127, 123, 117, 117, 117, 116, 121, 137, 171, 204, 276, 360, 428, 458, 487, 495, 449, 380, 288, 218, 189, 162, 145, 138, 132, 125, 133, 143, 143, 143, 147, 147, 149], [233, 218, 187, 179, 170, 163, 163, 169, 167, 154, 128, 117, 113, 116, 128, 160, 219, 322, 478, 647, 696, 630, 535, 414, 336, 284, 227, 189, 163, 146, 134, 127, 120, 125, 138, 144, 150, 160, 162, 154], [229, 215, 223, 260, 260, 232, 224, 245, 249, 211, 152, 126, 114, 114, 121, 144, 194, 283, 400, 516, 578, 560, 470, 360, 281, 226, 205, 175, 157, 143, 137, 133, 132, 136, 139, 144, 150, 160, 175, 169], [286, 260, 273, 342, 387, 361, 319, 306, 269, 224, 158, 129, 121, 119, 119, 131, 148, 174, 215, 254, 273, 286, 279, 244, 210, 190, 170, 156, 141, 135, 137, 140, 142, 141, 146, 154, 154, 166, 176, 185], [306, 320, 316, 377, 393, 364, 339, 319, 256, 200, 153, 126, 121, 116, 114, 120, 127, 128, 130, 143, 147, 155, 167, 162, 149, 143, 136, 131, 129, 133, 140, 139, 129, 137, 146, 150, 162, 169, 180, 187], [235, 260, 290, 326, 295, 267, 276, 277, 235, 185, 152, 134, 123, 117, 116, 114, 116, 120, 128, 137, 143, 137, 132, 127, 118, 116, 113, 117, 127, 129, 130, 129, 130, 146, 153, 151, 162, 162, 160, 150], [167, 174, 204, 233, 223, 202, 204, 217, 203, 161, 134, 123, 118, 115, 115, 118, 117, 112, 108, 113, 114, 117, 117, 121, 121, 124, 118, 123, 121, 119, 124, 129, 139, 156, 163, 154, 148, 142, 140, 135], [138, 145, 160, 174, 177, 165, 168, 174, 163, 135, 124, 118, 115, 112, 115, 116, 111, 106, 108, 107, 115, 106, 112, 116, 113, 116, 118, 116, 119, 120, 127, 135, 142, 173, 195, 196, 178, 151, 136, 137], [116, 123, 121, 130, 133, 135, 138, 141, 144, 130, 122, 117, 109, 104, 105, 109, 115, 116, 107, 105, 112, 114, 115, 115, 116, 119, 118, 119, 121, 125, 127, 137, 150, 195, 242, 230, 194, 159, 138, 136], [109, 112, 111, 119, 123, 124, 123, 123, 124, 122, 121, 117, 110, 104, 105, 108, 115, 114, 114, 113, 112, 112, 116, 116, 116, 117, 120, 122, 121, 125, 133, 141, 160, 204, 266, 259, 234, 205, 174, 160], [106, 107, 104, 109, 110, 112, 117, 127, 138, 128, 125, 124, 116, 107, 106, 107, 115, 113, 106, 108, 105, 108, 110, 108, 110, 123, 119, 120, 119, 129, 140, 145, 154, 195, 270, 309, 329, 329, 319, 290], [110, 111, 111, 110, 108, 111, 116, 128, 136, 133, 139, 139, 131, 123, 116, 114, 117, 114, 117, 115, 114, 112, 111, 110, 111, 115, 120, 122, 128, 132, 136, 148, 166, 200, 253, 286, 328, 367, 373, 347], [108, 102, 104, 102, 108, 111, 113, 116, 126, 154, 170, 163, 156, 138, 122, 122, 131, 128, 113, 112, 111, 110, 107, 111, 110, 104, 105, 110, 114, 122, 134, 151, 173, 201, 227, 218, 204, 211, 215, 208], [118, 119, 109, 108, 113, 112, 114, 129, 153, 158, 174, 190, 202, 182, 158, 146, 139, 129, 132, 122, 117, 109, 105, 110, 109, 107, 108, 109, 112, 114, 123, 137, 148, 189, 207, 189, 160, 146, 148, 145], [116, 123, 116, 113, 110, 109, 112, 117, 130, 155, 182, 222, 264, 257, 233, 201, 168, 158, 132, 127, 123, 118, 114, 113, 115, 113, 111, 107, 115, 122, 127, 134, 141, 163, 173, 164, 147, 136, 135, 120], [114, 116, 116, 110, 110, 109, 110, 111, 121, 151, 179, 214, 268, 295, 286, 253, 196, 169, 159, 149, 132, 124, 117, 112, 109, 104, 106, 108, 114, 116, 120, 134, 155, 156, 151, 140, 126, 120, 116, 119], [114, 113, 108, 108, 116, 113, 108, 108, 111, 127, 137, 155, 191, 217, 228, 219, 187, 167, 155, 142, 139, 131, 122, 122, 122, 119, 112, 107, 106, 107, 113, 121, 129, 135, 131, 124, 120, 121, 122, 130], [111, 106, 111, 114, 107, 106, 112, 117, 120, 119, 126, 139, 144, 146, 150, 155, 148, 140, 131, 132, 128, 126, 120, 113, 114, 121, 119, 112, 113, 117, 117, 119, 119, 117, 118, 122, 119, 124, 139, 156], [116, 114, 117, 121, 117, 110, 109, 113, 119, 114, 114, 131, 138, 134, 129, 126, 116, 116, 125, 126, 124, 121, 123, 121, 120, 121, 112, 108, 110, 115, 115, 114, 115, 112, 115, 114, 113, 121, 132, 140], [114, 110, 106, 109, 112, 112, 113, 113, 117, 118, 117, 125, 129, 122, 118, 117, 113, 110, 110, 120, 112, 113, 114, 112, 118, 118, 116, 107, 107, 108, 109, 109, 112, 114, 114, 113, 116, 120, 124, 124], [116, 112, 109, 107, 103, 108, 110, 109, 107, 108, 111, 120, 117, 114, 113, 113, 111, 108, 106, 106, 109, 114, 116, 118, 115, 113, 110, 113, 110, 107, 110, 117, 122, 116, 111, 114, 115, 114, 116, 115], [119, 112, 112, 109, 108, 106, 110, 112, 111, 109, 117, 122, 126, 122, 120, 119, 117, 120, 122, 119, 117, 118, 122, 121, 117, 118, 112, 110, 116, 115, 115, 119, 121, 120, 112, 114, 115, 117, 124, 122], [112, 111, 102, 98, 103, 110, 113, 113, 113, 108, 113, 115, 119, 114, 113, 110, 109, 112, 115, 116, 114, 122, 118, 115, 118, 119, 116, 121, 114, 105, 111, 125, 127, 127, 125, 122, 117, 116, 121, 124], [111, 113, 109, 103, 102, 105, 110, 104, 99, 103, 107, 104, 109, 112, 115, 112, 109, 108, 112, 115, 114, 110, 108, 110, 114, 120, 115, 113, 113, 119, 126, 138, 149, 147, 143, 133, 125, 121, 119, 114], [108, 113, 107, 103, 100, 99, 102, 101, 99, 101, 106, 114, 119, 122, 121, 116, 112, 107, 113, 115, 115, 110, 109, 113, 114, 114, 113, 117, 124, 136, 152, 175, 197, 209, 176, 156, 136, 121, 117, 119], [111, 112, 102, 102, 105, 102, 102, 105, 106, 105, 112, 125, 127, 130, 130, 131, 131, 120, 116, 115, 112, 114, 113, 109, 110, 118, 116, 125, 148, 175, 215, 260, 274, 286, 235, 176, 142, 126, 119, 117], [116, 111, 105, 104, 104, 105, 104, 108, 112, 106, 113, 118, 126, 140, 151, 154, 144, 140, 137, 135, 132, 127, 125, 121, 115, 108, 120, 140, 191, 263, 331, 363, 359, 301, 208, 164, 141, 130, 121, 116], [109, 113, 111, 118, 112, 106, 107, 108, 106, 105, 112, 116, 125, 147, 161, 168, 168, 163, 155, 157, 154, 148, 141, 132, 128, 120, 119, 124, 156, 209, 271, 317, 327, 277, 195, 157, 138, 127, 121, 124], [105, 101, 100, 106, 105, 104, 100, 98, 99, 103, 110, 120, 126, 141, 149, 152, 153, 158, 158, 154, 152, 150, 142, 133, 126, 127, 123, 117, 127, 152, 191, 230, 245, 224, 182, 148, 124, 116, 114, 117], [107, 100, 99, 102, 109, 107, 101, 100, 106, 108, 109, 118, 118, 123, 135, 142, 141, 135, 139, 147, 143, 134, 138, 139, 132, 125, 127, 123, 126, 135, 154, 173, 177, 170, 150, 132, 122, 117, 108, 104], [106, 99, 98, 100, 100, 103, 105, 105, 107, 100, 103, 110, 110, 113, 121, 125, 118, 118, 117, 113, 118, 122, 124, 125, 122, 129, 138, 128, 120, 122, 135, 146, 139, 138, 129, 122, 116, 115, 113, 113], [109, 106, 104, 99, 103, 107, 107, 106, 104, 104, 104, 109, 113, 116, 117, 117, 120, 117, 113, 122, 123, 121, 122, 119, 121, 143, 136, 125, 125, 126, 125, 126, 125, 124, 119, 112, 107, 109, 111, 113], [110, 108, 110, 111, 113, 116, 109, 103, 103, 104, 106, 108, 110, 113, 114, 113, 119, 123, 126, 117, 112, 117, 122, 118, 121, 135, 126, 118, 117, 117, 118, 119, 118, 108, 111, 124, 128, 120, 119, 119], [107, 106, 108, 109, 111, 111, 109, 113, 113, 105, 103, 104, 107, 108, 108, 109, 109, 111, 114, 116, 120, 124, 126, 122, 117, 119, 121, 131, 128, 127, 125, 120, 113, 111, 114, 118, 115, 111, 113, 113], [112, 107, 106, 111, 116, 119, 115, 111, 107, 104, 104, 101, 102, 104, 105, 103, 105, 105, 108, 115, 115, 116, 118, 121, 117, 117, 120, 120, 119, 119, 119, 119, 117, 118, 114, 110, 109, 108, 110, 115], [116, 115, 116, 120, 127, 124, 118, 111, 105, 106, 105, 111, 108, 107, 107, 108, 106, 106, 114, 124, 124, 127, 125, 125, 123, 122, 123, 121, 123, 122, 117, 118, 120, 118, 115, 115, 112, 111, 119, 135], [126, 133, 135, 146, 150, 137, 122, 115, 114, 114, 113, 113, 106, 108, 110, 107, 100, 97, 106, 116, 121, 131, 132, 134, 126, 124, 117, 113, 113, 118, 117, 117, 114, 118, 114, 118, 119, 115, 124, 136]]
  in  "plot range":dbl=40.0
  in  "marker":u32(colorbox)=16448250
  in  "point radius":i16=2
  in  "mag":dbl=4.0 format="%_2g"
  in  "color":T6={"color array"=[255, 6618880, 16711680, 16776960, 16711680, 16711935, 16448250, 16448250], "num of colors"=3, "max"=1.4999999999999996, "min"=0.5} {"min" step=0.01 format="%_2f"; "max" step=0.1 format="%_3f"}
  in  "pixel center":cluster{"horizontal":i16, "vertical":i16}={"horizontal"=45, "vertical"=45}
  out "FWHMx":picture
  out "FWHMy [um]":dbl=0.5057156254984324
  out "FWHMx [um]":dbl=1.191696488335398
  out "y2":dbl[][](graph)=[[200.22199072102043, 205.97930360182497, 264.8716279352452, 483.49629992621266, 699.0320064563291, 553.8325759270325, 301.05449468829465, 211.62523826650454], [252.0, 259.0, 318.0, 458.0, 696.0, 578.0, 273.0, 147.0]]
  out "x2":dbl[][](graph)=[[135.31989834032066, 135.6435029385883, 136.96695794691126, 141.5127929577792, 154.58161980214248, 185.86900506030582, 247.74859251728947, 347.49262892090496, 475.1797494553423, 597.4426586112784, 668.752491740053, 658.0434259291361, 570.1645615499507, 442.40455579204286, 319.406172596063, 228.98110084070453, 175.7470978211116, 150.09974163165543, 139.86767893611494, 136.46336148348794], [128.0, 117.0, 113.0, 116.0, 128.0, 160.0, 219.0, 322.0, 478.0, 647.0, 696.0, 630.0, 535.0, 414.0, 336.0, 284.0, 227.0, 189.0, 163.0, 146.0]]
  in  "fitting range x":dbl=20.0
  in  "n of avg":dbl=1.0
  in  "raw object index":i32(slide) min=0 max=38 scale=0.0..38.0
  in  "Stop":bool
  in  "Ny2":i32=300
  in  "Nz2":i32=100
  out "pixsize@spl [um]":dbl=0.20478890989287965
  in  "magnification":dbl=31.74 format="%#_13g"
  in  "pixel size [um]":dbl=6.5 format="%#_13g"
  in  "intensity":dbl=500.0 format="%#_13g"
  in  "noise":dbl=1.0000000000000002 format="%0.2f"
  out "xy MIP":i32[][](graph)
  in  "# of beads":i32=100
  out "x":cluster{dbl[], dbl[]}[](graph)=[{[-2.1249257347652626, -1.920136824872383, -1.7153479149795032, -1.5105590050866236, -1.3057700951937439, -1.1009811853008644, -0.8961922754079846, -0.6914033655151051, -0.4866144556222254, -0.2818255457293457, -0.07703663583646606, 0.1277522740564136, 0.3325411839492932, 0.5373300938421729, 0.7421190037350526, 0.9469079136279321, 1.1516968235208118, 1.3564857334136915, 1.5612746433065712, 1.7660635531994509], [28.0, 17.0, 13.0, 16.0, 28.0, 60.0, 119.0, 222.0, 378.0, 547.0, 596.0, 530.0, 435.0, 314.0, 236.0, 184.0, 127.0, 89.0, 63.0, 46.0]}, {array[1000 elements], array[1000 elements]}]
  out "y":cluster{dbl[], dbl[]}[](graph)=[{[-0.8441118813908094, -0.6393229714979297, -0.4345340616050501, -0.22974515171217044, -0.0249562418192908, 0.17983266807358886, 0.3846215779664685, 0.5894104878593481], [152.0, 159.0, 218.0, 358.0, 596.0, 478.0, 173.0, 47.0]}, {array[1000 elements], array[1000 elements]}]
  out "z":cluster{dbl[], dbl[]}[](graph)=[{[-3.171978904499398, -2.967189994606518, -2.7624010847136384, -2.557612174820759, -2.352823264927879, -2.1480343550349996, -1.9432454451421197, -1.7384565352492403, -1.5336676253563606, -1.328878715463481, -1.1240898055706012, -0.9193008956777216, -0.7145119857848419, -0.5097230758919623, -0.30493416599908263, -0.10014525610620297, 0.10464365378667669, 0.30943256367955635, 0.514221473572436, 0.7190103834653157, 0.9237992933581953, 1.128588203251075, 1.3333771131439547, 1.5381660230368341, 1.7429549329297138, 1.9477438428225935, 2.1525327527154734, 2.357321662608353, 2.5621105725012323, 2.766899482394112], [40.0, 42.0, 46.0, 60.0, 73.0, 95.0, 111.0, 138.0, 171.0, 206.0, 239.0, 285.0, 369.0, 454.0, 523.0, 596.0, 578.0, 500.0, 455.0, 390.0, 317.0, 255.0, 182.0, 136.0, 105.0, 79.0, 63.0, 56.0, 56.0, 61.0]}, {array[1000 elements], array[1000 elements]}]
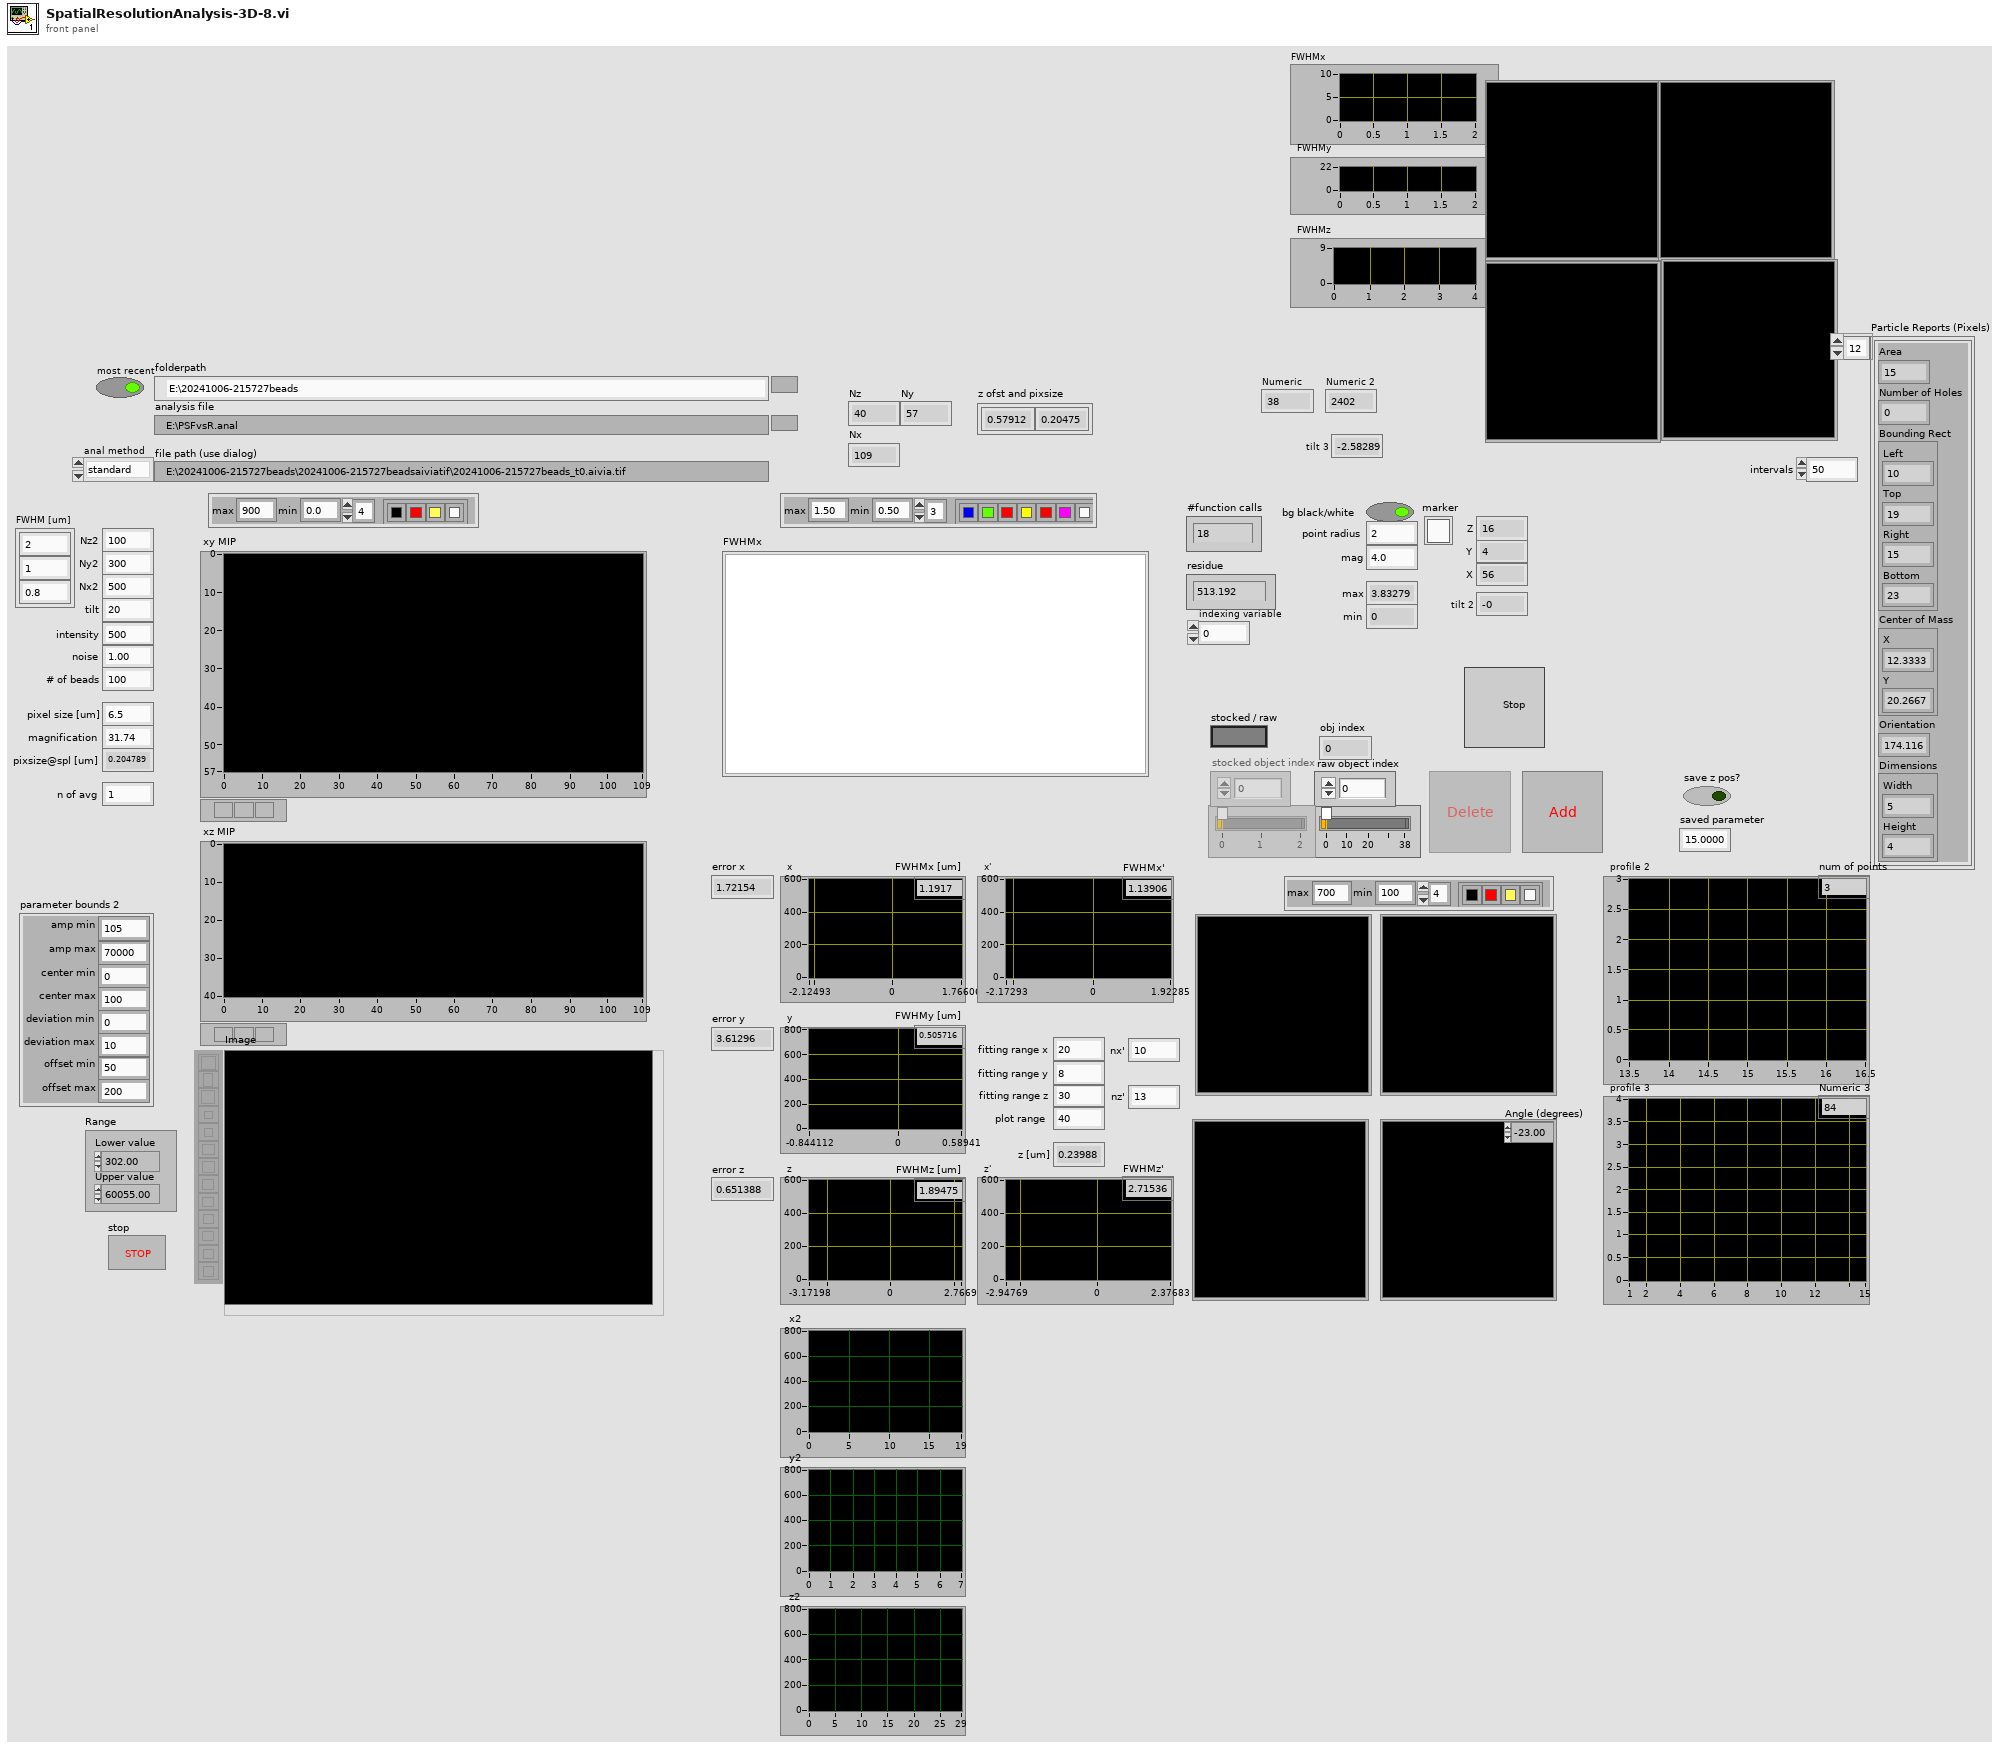
[diagram p1: front panel]
types:
  T1 = typedef "IMAQ Image.ctl" = refnum<image>
  T2 = cluster{"Area":dbl, "Number of Holes":dbl, "Bounding Rect":cluster{"Left":dbl, "Top":dbl, "Right":dbl, "Bottom":dbl}, "Center of Mass":cluster{"X":dbl, "Y":dbl}, "Orientation":dbl, "Dimensions":cluster{"Width":dbl, "Height":dbl}}[]
  T3 = enum16{"standard", "2D tilted Gaussian fit for zx"}
  T4 = cluster{"X Values":dbl[], "Histogram: h(x)":i32[]}
  T5 = cluster{"amp min":dbl, "amp max":dbl, "center min":dbl, "center max":dbl, "deviation min":dbl, "deviation max":dbl, "offset min":dbl, "offset max":dbl}
  T6 = cluster{"color array":u32[], "num of colors":i32, "max":dbl, "min":dbl}
  T7 = typedef "Image Type" = u32
  T8 = enum16{"open", "replace", "create", "open or create", "replace or create", "replace or create with confirmation"}
  T9 = cluster{"z [um]":dbl, "Particle Report":cluster{"Area":dbl, "Number of Holes":dbl, "Bounding Rect":cluster{"Left":dbl, "Top":dbl, "Right":dbl, "Bottom":dbl}, "Center of Mass":cluster{"X":dbl, "Y":dbl}, "Orientation":dbl, "Dimensions":cluster{"Width":dbl, "Height":dbl}}, "yx":u16[][], "zx":u16[][], "zy":u16[][], "filepath":string, "FWHMx'":dbl, "x' profiles":cluster{"fit x":dbl[], "fit y":dbl[]}[], "FWHMz'":dbl, "z' profiles":cluster{"fit x":dbl[], "fit y":dbl[]}[], "input cluster":cluster{"x profile":dbl[][], "y profile":dbl[][], "z profile":dbl[][], "FWHMx[um]":dbl, "FWHMy[um]":dbl, "FWHMz[um]":dbl, "z pos":i32, "tilt":dbl, "error x":dbl, "error y":dbl, "error z":dbl, "error max":dbl, "coeffs x":dbl[], "coeffs y":dbl[], "coeffs z":dbl[], "profiles x":cluster{dbl[], dbl[]}[], "profiles y":cluster{dbl[], dbl[]}[], "profiles z":cluster{dbl[], dbl[]}[], "x pos":i32, "y pos":i32}}
  T10 = cluster{"z [um]":dbl, "Particle Report":cluster{"Area":dbl, "Number of Holes":dbl, "Bounding Rect":cluster{"Left":dbl, "Top":dbl, "Right":dbl, "Bottom":dbl}, "Center of Mass":cluster{"X":dbl, "Y":dbl}, "Orientation":dbl, "Dimensions":cluster{"Width":dbl, "Height":dbl}}, "yx":u16[][], "zx":u16[][], "zy":u16[][], "filepath":string, "FWHMx'":dbl, "x' profiles":cluster{"fit x":dbl[], "fit y":dbl[]}[], "FWHMz'":dbl, "z' profiles":cluster{"fit x":dbl[], "fit y":dbl[]}[], "input cluster":cluster{"x profile":dbl[][], "y profile":dbl[][], "z profile":dbl[][], "FWHMx[um]":dbl, "FWHMy[um]":dbl, "FWHMz[um]":dbl, "z pos":i32, "tilt":dbl, "error x":dbl, "error y":dbl, "error z":dbl, "error max":dbl, "coeffs x":dbl[], "coeffs y":dbl[], "coeffs z":dbl[], "profiles x":cluster{dbl[], dbl[]}[], "profiles y":cluster{dbl[], dbl[]}[], "profiles z":cluster{dbl[], dbl[]}[], "x pos":i32, "y pos":i32}}[]
  T11 = cluster{"Width":u16, "Style":enum32{"Solid", "Dash", "Dot", "DashDot", "DashDotDot"}}
  T12 = typedef "LVBoundsTypeDef.ctl" = cluster{"Width":u32, "Height":u32}
  T13 = cluster{"x profile":dbl[][], "y profile":dbl[][], "z profile":dbl[][], "FWHMx[um]":dbl, "FWHMy[um]":dbl, "FWHMz[um]":dbl, "z pos":i32, "tilt":dbl, "error x":dbl, "error y":dbl, "error z":dbl, "error max":dbl, "coeffs x":dbl[], "coeffs y":dbl[], "coeffs z":dbl[], "profiles x":cluster{dbl[], dbl[]}[], "profiles y":cluster{dbl[], dbl[]}[], "profiles z":cluster{dbl[], dbl[]}[], "x pos":i32, "y pos":i32}
  T14 = enum8{"Enabled", "Disabled", "Disabled and Grayed Out"}
  T15 = cluster{"parameter bounds 2":cluster{"amp min":dbl, "amp max":dbl, "center min":dbl, "center max":dbl, "deviation min":dbl, "deviation max":dbl, "offset min":dbl, "offset max":dbl}, "anal method":enum16{"standard", "2D tilted Gaussian fit for zx"}, "fitting range x":dbl, "fitting range y":dbl, "fitting range z":dbl, "n of avg":dbl}
  T16 = cluster{"Area":dbl, "Number of Holes":dbl, "Bounding Rect":cluster{"Left":dbl, "Top":dbl, "Right":dbl, "Bottom":dbl}, "Center of Mass":cluster{"X":dbl, "Y":dbl}, "Orientation":dbl, "Dimensions":cluster{"Width":dbl, "Height":dbl}}
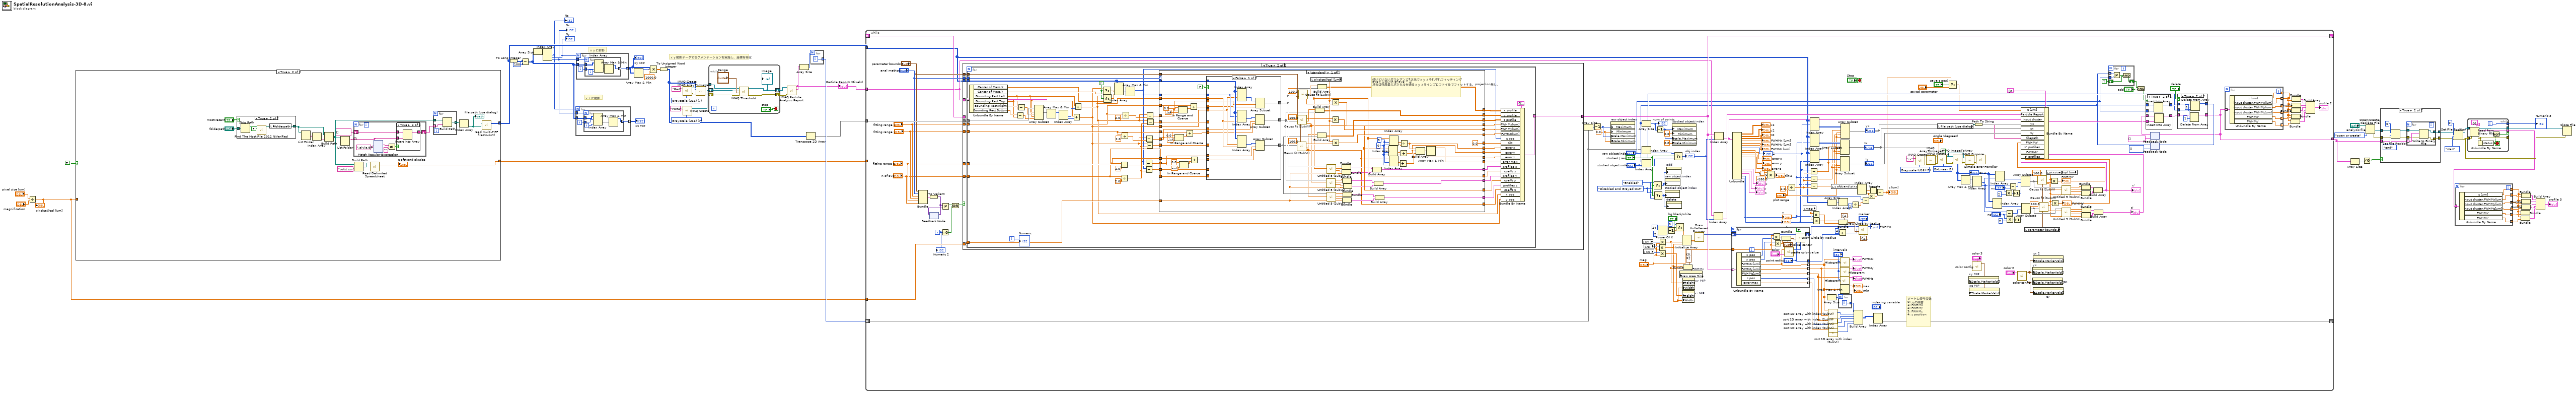
[diagram p0: block diagram]
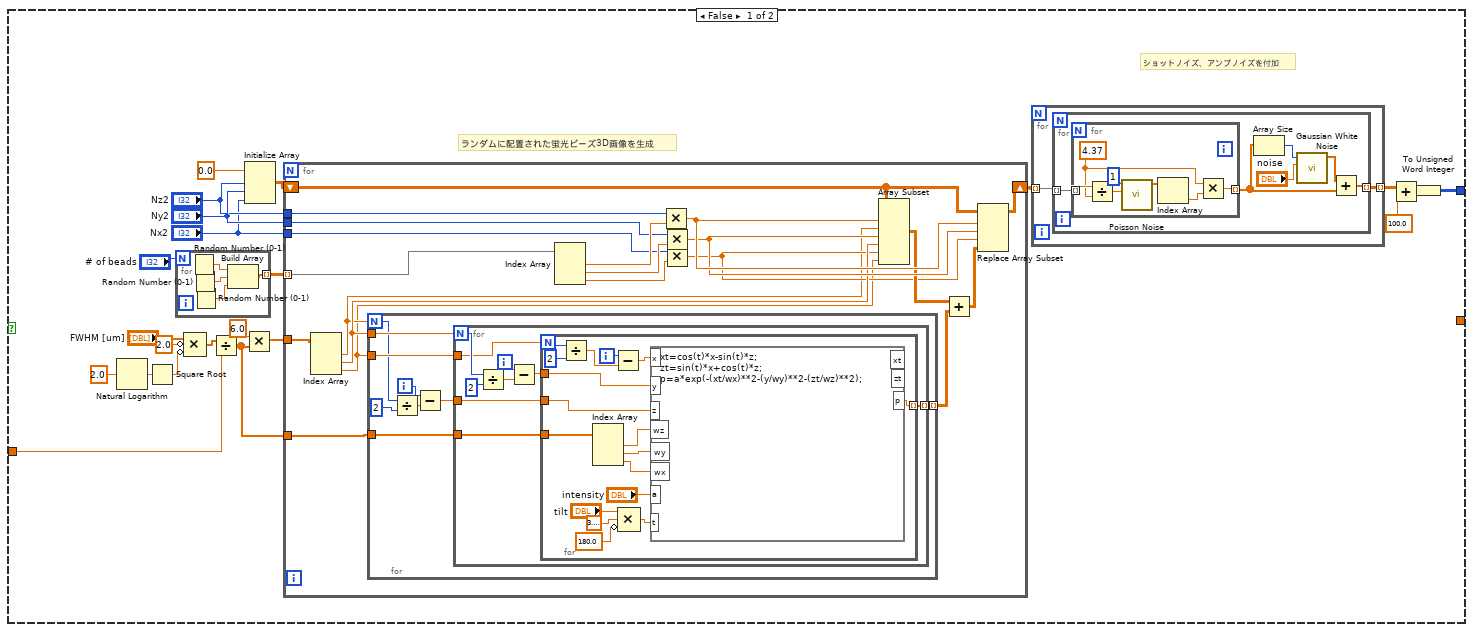
[diagram p3: hidden frame]
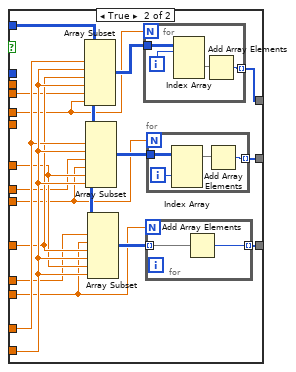
[diagram p9: hidden frame]
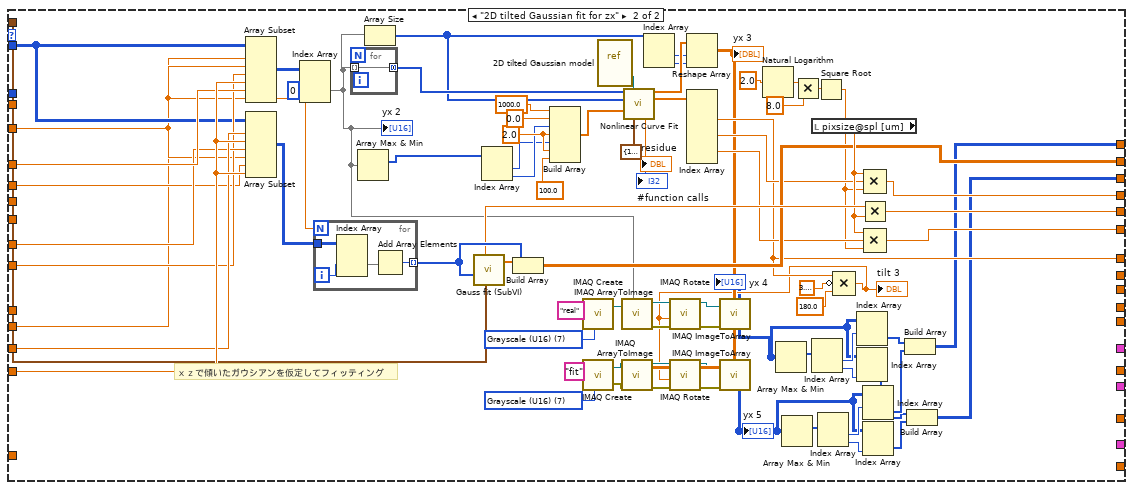
[diagram p10: hidden frame]
diagram:
  w3 = T7 7 items=["Grayscale (U8)", "Grayscale (I16)", "Grayscale (SGL)", "Complex (CSG)", "RGB (U32)", "HSL (U32)", "RGB (U64)", "Grayscale (U16)"] ("Image Type")
  w42 = T7 7 items=["Grayscale (U8)", "Grayscale (I16)", "Grayscale (SGL)", "Complex (CSG)", "RGB (U32)", "HSL (U32)", "RGB (U64)", "Grayscale (U16)"] ("Image Type")
  # "ｘｙ射影データでセグメンテーションを実施し、座標を特定"
  # "ｘｚに射影"
  # "ｘｙに射影"
  n1 = Divide(x="pixel size [um]", y="magnification") -> (x/y=w46:dbl)
  "pixsize@spl [um]" <- w46
  n2 = case shown="True" TRUE ("open img file") {
    tunnel: [w67 w173] -> w48
    tunnel: w46 -> [w63 _]
    tunnel: [_ w159] -> w38
    frame False {
      # "ショットノイズ、アンプノイズを付加"
      # "ランダムに配置された蛍光ビーズ3D画像を生成"
      n3 = Natural Logarithm(1:2.0 ("x")) -> (0:w65:dbl)
      n4 = Square Root(x=w65) -> (sqrt(x)=w64:dbl)
      n5 = for {
        N: "# of beads" -> [_]
        tunnel: [w156] -> w83 mode=indexing
        n6 = Random Number (0-1)() -> (number: 0 to 1=w158:dbl)
        n7 = Random Number (0-1)() -> (number: 0 to 1=w157:dbl)
        n8 = Random Number (0-1)() -> (number: 0 to 1=w155:dbl)
        n9 = Build Array(w158, w157, w155) -> (w156:dbl[])
      }
      n10 = Compound Arithmetic op=MULTIPLY("FWHM [um]", invert 2.0 ("y"), invert w64) -> (w80:dbl[])
      n11 = Divide(x=w80, y=w63) -> (x/y=w72:dbl[])
      n12 = Multiply(x=6.0, y=w72) -> (x*y=w74:dbl[])
      n13 = Initialize Array(0.0 ("element"), "Nz2", "Ny2", "Nx2") -> (w76:dbl[][][])
      n14 = for {
        tunnel: w83 -> [w118] mode=indexing
        tunnel: "Nz2" -> [w119]
        tunnel: "Ny2" -> [w115]
        shift-right: [w114] -> w73
        shift-left: w76 -> [w112]
        tunnel: w74 -> [w104]
        tunnel: w72 -> [w113]
        tunnel: "Nx2" -> [w106]
        n15 = Index Array(array=w104) -> (element #1=w101:dbl, element #2=w103:dbl, element #3=w100:dbl)  [unwired: 3 in]
        n16 = for {
          N: w101 -> [w123]
          tunnel: w113 -> [w128]
          tunnel: [w127] -> w109 mode=indexing
          tunnel: w100 -> [w126]
          tunnel: w103 -> [w125]
          i -> [w122]
          n17 = Divide(x=w123, y=2) -> (x/y=w121:dbl)
          n18 = Subtract(x=w122, y=w121) -> (x-y=w120:dbl)
          n19 = for {
            N: w125 -> [w136]
            tunnel: [w137] -> w127 mode=indexing
            tunnel: w128 -> [w131]
            tunnel: w126 -> [w130]
            tunnel: w120 -> [w129]
            i -> [w134]
            n20 = Divide(x=w136, y=2) -> (x/y=w133:dbl)
            n21 = Subtract(x=w134, y=w133) -> (x-y=w132:dbl)
            n22 = for {
              N: w130 -> [w144]
              tunnel: w132 -> [w154]
              tunnel: [w152] -> w137 mode=indexing
              tunnel: w131 -> [w149]
              tunnel: w129 -> [w142]
              i -> [w151]
              n23 = Divide(x=w144, y=2) -> (x/y=w143:dbl)
              n24 = Index Array(array=w149) -> (element #1=w148:dbl, element #2=w147:dbl, element #3=w146:dbl)  [unwired: 3 in]
              n25 = Subtract(x=w151, y=w143) -> (x-y=w150:dbl)
              n26 = Compound Arithmetic op=MULTIPLY("tilt", 3.141592653589793, invert 180.0 ("value")) -> (w140:dbl)
              n27 = formula code="xt=cos(t)*x-sin(t)*z;\nzt=sin(t)*x+cos(t)*z;\np=a*exp(-(xt/wx)**2-(y/wy)**2-(zt/wz)**2);"("x"=w150, "y"=w154, "wz"=w148, "a"="intensity", "wy"=w147, "wx"=w146, "z"=w142, "t"=w140) -> ("p"=w152:dbl)  [unwired: 2 out]
            }
          }
        }
        n28 = Index Array(array=w118) -> (element #1=w117:dbl, element #2=w116:dbl, element #3=w105:dbl)  [unwired: 3 in]
        n29 = Multiply(x=w119, y=w117) -> (x*y=w111:dbl)
        n30 = Multiply(x=w115, y=w116) -> (x*y=w110:dbl)
        n31 = Multiply(x=w106, y=w105) -> (x*y=w102:dbl)
        n32 = Array Subset(array=w112, index (dim 0)=w111, length (dim 0)=w101, index (dim 1)=w110, length (dim 1)=w103, index (dim 2)=w102, length (dim 2)=w100) -> (w108:dbl[][][])
        n33 = Add(x=w108, y=w109) -> (x+y=w107:dbl[][][])
        n34 = Replace Array Subset(array=w112, new element=w107, index (dim 0)=w111, index (dim 1)=w110, index (dim 2)=w102) -> (w114:dbl[][][])
      }
      n35 = for {
        tunnel: [w86] -> w82 mode=indexing
        tunnel: w73 -> [w85] mode=indexing
        n36 = for {
          tunnel: w85 -> [w89] mode=indexing
          tunnel: [w90] -> w86 mode=indexing
          n37 = for {
            tunnel: w89 -> [w97] mode=indexing
            tunnel: [w94] -> w88 mode=indexing
            w95 = 4.37
            n38 = Divide(x=w97, y=w95) -> (x/y=w93:dbl)
            n39 = call <vilib>:"Poisson Noise.vi"("mean"=w93, "samples"=1) -> ("poisson noise"=w98:dbl[])  [unwired: 8 in, 1 out]
            n40 = Index Array(array=w98) -> (element=w96:dbl)  [unwired: 1 in]
            n41 = Multiply(x=w95, y=w96) -> (x*y=w94:dbl)
          }
          n42 = Array Size(array=w88) -> (size(s)=w92:i32)
          n43 = call <vilib>:"Gaussian White Noise.vi"("standard deviation"="noise", "samples"=w92) -> ("Gaussian noise pattern"=w91:dbl[])  [unwired: 8 in, 1 out]
          n44 = Add(x=w91, y=w88) -> (x+y=w90:dbl[])
        }
      }
      n45 = Add(x=w82, y=100.0) -> (x+y=w68:dbl[][][])
      n46 = To Unsigned Word Integer(number=w68) -> (unsigned 16bit integer=w67:u16[][][])
    }
    frame True {
      n47 = case shown="True" "most recent" {
        tunnel: "folderpath" -> [w305 w308]
        tunnel: [w305 w306] -> w167
        frame False {
        }
        frame True {
          n48 = Strip Path(path=w308) -> (stripped path=w307:path)  [unwired: 1 out]
          n49 = call "Find The Most File 2012 NIVerified.vi"("file(T)/folder(F)"=FALSE, "Folder Path In"=w307) -> ("File Path Out"=w306:path)  [unwired: 8 in, 1 out]
          n50 = local write "folderpath"(w306) -> ()
        }
      }
      n51 = List Folder(path=w167) -> (folder names=w168:string[])  [unwired: 3 in, 3 out]
      n52 = Index Array(array=w168) -> (element=w166:string)  [unwired: 1 in]
      n53 = Build Path(base path=w167, name or relative path=w166) -> (appended path=w164:path)
      n54 = List Folder(path=w164) -> (filenames=w165:string[])  [unwired: 3 in, 3 out]
      n55 = for {
        tunnel: w165 -> [w175] mode=indexing
        shift-right: [w177] -> w169
        shift-left: string[] [] -> [w178]
        n56 = xnode "Match Regular Expression"("input string"=w175, "regular expression"=".aivia.tif") -> ("whole match"=w179:string)  [unwired: 4 in, 4 out]
        n57 = Not Equal?(x=w179, y="") -> (x != y?=w176:bool)
        n58 = case shown="True" w176 {
          tunnel: w178 -> [w181 w184]
          tunnel: [w181 w183] -> w177
          tunnel: w175 -> [_ w182]
          frame False {
          }
          frame True {
            n59 = Insert Into Array(array=w184, new element=w182) -> (w183:string[])  [unwired: 1 in]
          }
        }
      }
      n60 = Build Path(base path=w164, name or relative path="zofst.csv" ("regular expression")) -> (appended path=w162:path)
      n61 = call-poly <vilib>:"Read Delimited Spreadsheet.vi"("file path (dialog if empty)"=w162) -> ("first row"=w159:dbl[])  [unwired: 9 in, 5 out]
      "z ofst and pixsize" <- w159
      n62 = for {
        tunnel: w169 -> [w304] mode=indexing
        tunnel: w164 -> [w303]
        tunnel: [w302] -> w161 mode=indexing
        n63 = Build Path(base path=w303, name or relative path=w304) -> (appended path=w302:path)
      }
      n64 = Index Array(array=w161) -> (element=w160:path)  [unwired: 1 in]
      "file path (use dialog)" <- w160
      n65 = call "read multi-TIFF files(subVI).vi"("file path (use dialog)"=w160) -> ("image data"=w173:u16[][][])  [unwired: 2 in]
    }
  }
  n66 = To Long Integer(number=w48) -> (32bit integer=w61:i32[][][])
  n67 = Subtract(x=w61, y=100) -> (x-y=w56:i32[][][])
  n68 = Array Size(array=w56) -> (size(s)=w62:i32[])
  n69 = Index Array(array=w62) -> (element #1=w40:i32, element #2=w41:i32, element #3=w39:i32)  [unwired: 3 in]
  "Nz" <- w40
  "Ny" <- w41
  "Nx" <- w39
  n70 = for {
    N: w40 -> [_]
    tunnel: w56 -> [w313]
    tunnel: [w312] -> w55 mode=indexing
    tunnel: w39 -> [w310]
    i -> [w311]
    n71 = for {
      N: w310 -> [_]
      tunnel: w313 -> [w318]
      tunnel: [w315] -> w312 mode=indexing
      tunnel: w311 -> [w317]
      i -> [w316]
      n72 = Index Array(array=w318, index (dim 0)=w317, index (dim 2)=w316) -> (element=w314:i32[])  [unwired: 1 in]
      n73 = Array Max & Min(array=w314) -> (max value=w315:i32)  [unwired: 3 out]
    }
  }
  "xz MIP" <- w55
  n74 = for {
    N: w41 -> [_]
    tunnel: w56 -> [w322]
    tunnel: [w321] -> w29 mode=indexing
    tunnel: w39 -> [w319]
    i -> [w320]
    n75 = for {
      N: w319 -> [_]
      tunnel: w322 -> [w327]
      tunnel: [w323] -> w321 mode=indexing
      tunnel: w320 -> [w325]
      i -> [w324]
      n76 = Index Array(array=w327, index (dim 1)=w325, index (dim 2)=w324) -> (element=w326:i32[])  [unwired: 1 in]
      n77 = Array Max & Min(array=w326) -> (max value=w323:i32)  [unwired: 3 out]
    }
  }
  "xy MIP" <- w29
  n78 = Array Max & Min(array=w29) -> (max value=w59:i32)  [unwired: 3 out]
  n79 = Compound Arithmetic op=MULTIPLY(w29, invert w59, 1000.0 ("value")) -> (w58:dbl[][])
  n80 = To Unsigned Word Integer(number=w58) -> (unsigned 16bit integer=w30:u16[][])
  n81 = call "IMAQ Create"("Image Name"="Part", "Image Type"=w42) -> ("New Image"=w44:T1, "error out"=w43:errorcluster)  [unwired: 3 in]
  n82 = call "IMAQ Create"("Image Name"="Part2", "Image Type"=w3) -> ("New Image"=w2:T1)  [unwired: 3 in, 1 out]
  n83 = call "IMAQ ArrayToImage"("Image Pixels (U16)"=w30, "error in (no error)"=w43, "Image"=w44) -> ("error out"=w33:errorcluster, "Image Out"=w1:T1)  [unwired: 7 in]
  n84 = while {
    shift-right: [w333] -> w32
    shift-left: w2 -> [w328]
    shift-right: [w332] -> w31
    shift-left: w33 -> [w334]
    tunnel: w1 -> [w329]
    stop <- "stop" stop-if-true
    n85 = call "IMAQ Threshold"("error in (no error)"=w334, "Range"="Range", "Image Dst"=w328, "Image Src"=w329) -> ("error out"=w332:errorcluster, "Image Dst Out"=w333:T1)  [unwired: 6 in]
    "Image" <- w333
  }
  n86 = call "IMAQ Particle Analysis Report"("error in (no error)"=w31, "Image"=w32) -> ("Particle Reports (Pixels)"=w49:T2)  [unwired: 4 in, 5 out]
  "Particle Reports (Pixels)" <- w49
  n87 = Array Size(array=w49) -> (size(s)=w54:i32)
  n88 = Transpose 2D Array(2D array=w30) -> (transposed array=w47:u16[][])
  n89 = for {
    N: w54 -> [_]
    tunnel: [w335] -> w53 mode=indexing
    i -> [w335]
  }
  n90 = while {
    tunnel: w48 -> [w454]
    shift-right: [w504] -> _
    shift-left: w53 -> [w347]
    tunnel: w49 -> [w466]
    tunnel: w47 -> [w488]
    tunnel: w46 -> [w487]
    shift-right: [w473] -> _
    shift-left: _ -> [w472]
    tunnel: w38 -> [_]
    tunnel: [w363] -> w7
    i -> [w476]
    stop <- "Stop" stop-if-true
    w344 = 0.0 ("Scale.Range:Minimum")
    w367 = T14."Disabled and Grayed Out" ("Disabled")
    w366 = T14."Enabled" ("Disabled")
    w431 = 1 items=["Zero Order", "Bi-Linear"] ("Interpolation Type")
    w438 = T7 7 items=["Grayscale (U8)", "Grayscale (I16)", "Grayscale (SGL)", "Complex (CSG)", "RGB (U32)", "HSL (U32)", "RGB (U64)", "Grayscale (U16)"] ("Image Type")
    # "ソートに使う変数\n0: 元の順番\n1: FWHMx\n2: FWHMy\n3: FWHMz\n4: z position"
    n91 = Bundle("parameter bounds 2"="parameter bounds 2", "anal method"="anal method", "fitting range x"="fitting range x", "fitting range y"="fitting range y", "fitting range z"="fitting range z", "n of avg"="n of avg") -> (w480:T15)  [unwired: 1 in]
    n92 = To Variant(anything=w480) -> (Variant=w479:variant)
    n93 = feedback-in #1(w479) -> ()
    n94 = feedback #1() -> (w478:variant)  [unwired: 1 in]
    n95 = Equal To 0?(x=w476) -> (x = 0?=w474:bool)
    n96 = Not Equal?(x=w479, y=w478) -> (x != y?=w477:bool)
    n97 = Or(x=w477, y=w474) -> (x .or. y?=w475:bool)
    n98 = case shown="True" w475 {
      tunnel: [w589 w600] -> w473
      tunnel: w466 -> [_ w599]
      tunnel: w454 -> [_ w598]
      tunnel: w488 -> [_ w597]
      tunnel: w487 -> [_ w596]
      tunnel: "parameter bounds 2" -> [_ w595]
      tunnel: "anal method" -> [_ w594]
      tunnel: "fitting range x" -> [_ w593]
      tunnel: "fitting range y" -> [_ w592]
      tunnel: "fitting range z" -> [_ w591]
      tunnel: "n of avg" -> [_ w590]
      tunnel: w472 -> [w589 _]
      frame False {
      }
      frame True {
        n99 = for {
          tunnel: w598 -> [w652]
          tunnel: w599 -> [w663] mode=indexing
          tunnel: [w645] -> w600 mode=indexing
          tunnel: w597 -> [w636]
          tunnel: w596 -> [w620]
          tunnel: w594 -> [w615]
          tunnel: w595 -> [w614]
          tunnel: w592 -> [w613]
          tunnel: w591 -> [w612]
          tunnel: w593 -> [w611]
          tunnel: w590 -> [w610]
          i -> [w643]
          w623 = TRUE ("xy max pos(T)/center of mass(F)")
          n100 = Unbundle By Name(w663) -> ("Center of Mass.X"=w625:dbl, "Center of Mass.Y"=w627:dbl, "Bounding Rect.Left"=w631:dbl, "Bounding Rect.Top"=w629:dbl, "Bounding Rect.Right"=w638:dbl, "Bounding Rect.Bottom"=w637:dbl)
          n101 = Subtract(x=w637, y=w629) -> (x-y=w634:dbl)
          n102 = Subtract(x=w638, y=w631) -> (x-y=w635:dbl)
          n103 = Array Subset(array=w636, index (row)=w631, length (row)=w635, index (col)=w629, length (col)=w634) -> (w633:u16[][])
          n104 = Array Max & Min(array=w633) -> (max index (indices)=w632:i32[])  [unwired: 3 out]
          n105 = Index Array(array=w632) -> (element #1=w630:i32, element #2=w628:i32)  [unwired: 2 in]
          n106 = Add(x=w629, y=w628) -> (x+y=w601:dbl)
          n107 = Add(x=w631, y=w630) -> (x+y=w602:dbl)
          n108 = Select(t=w601, s=w623, f=w627) -> (s? t:f=w626:dbl)
          n109 = Select(t=w602, s=w623, f=w625) -> (s? t:f=w624:dbl)
          n110 = Index Array(array=w652, index (dim 1)=w626, index (dim 2)=w624) -> (element=w660:u16[])  [unwired: 1 in]
          n111 = Divide(x=w612, y=2.0) -> (x/y=w619:dbl)
          n112 = Divide(x=w610, y=2.0) -> (x/y=w659:dbl)
          n113 = Divide(x=w613, y=2.0) -> (x/y=w616:dbl)
          n114 = Divide(x=w611, y=2.0) -> (x/y=w621:dbl)
          n115 = Array Max & Min(array=w660) -> (max index (indices)=w609:i32)  [unwired: 3 out]
          n116 = Subtract(x=w609, y=w619) -> (x-y=w657:dbl)
          n117 = Subtract(x=w609, y=w659) -> (x-y=w656:dbl)
          n118 = Subtract(x=w601, y=w616) -> (x-y=w655:dbl)
          n119 = Subtract(x=w601, y=w659) -> (x-y=w654:dbl)
          n120 = Subtract(x=w602, y=w621) -> (x-y=w658:dbl)
          n121 = Subtract(x=w602, y=w659) -> (x-y=w653:dbl)
          n122 = case shown="\"standard\"" w615 {
            tunnel: w610 -> [w749 w873]
            tunnel: w658 -> [w703 w872]
            tunnel: w657 -> [w705 w841]
            tunnel: w656 -> [w748 w871]
            tunnel: w655 -> [w704 w870]
            tunnel: w654 -> [w747 w869]
            tunnel: w653 -> [w746 w868]
            tunnel: w652 -> [w745 w867]
            tunnel: w611 -> [w713 w857]
            tunnel: [w738 w794] -> w651
            tunnel: [w737 w844] -> w650
            tunnel: [w736 w793] -> w649
            tunnel: [w735 w860] -> w648
            tunnel: [w734 w859] -> w647
            tunnel: [w733 w858] -> w646
            tunnel: [0.0 ("tilt") w821] -> w644
            tunnel: w614 -> [w731 w846]
            tunnel: [w720 _] -> w642
            tunnel: [w719 _] -> w641
            tunnel: [w718 _] -> w640
            tunnel: [w728 _] -> w639
            tunnel: w612 -> [w717 _]
            tunnel: w620 -> [w684 _]
            tunnel: [w682 _] -> w618
            tunnel: w613 -> [w700 _]
            tunnel: [w681 _] -> w606
            tunnel: [w664 _] -> w604
            tunnel: w609 -> [w695 _]
            tunnel: w602 -> [w694 _]
            tunnel: w601 -> [w693 _]
            tunnel: [w667 _] -> w608
            tunnel: [w666 _] -> w607
            tunnel: [w665 _] -> w605
            frame "standard" {
              w727 = 0 ("index")
              w730 = 3 ("index")
              # "傾いていないガウシアンで1次元でｘｙｚそれぞれフィッティング\navgとらない(n of avg = 1) 場合は強度最大ボクセルを通るｘｙｚラインプロファイルでフィットする。projection無し。"
              n123 = In Range and Coerce(upper limit=0.0, x=w704, lower limit=-inf) -> (coerced(x)=w699:dbl)  [unwired: 1 out]
              n124 = In Range and Coerce(upper limit=0.0, x=w703, lower limit=-inf) -> (coerced(x)=w701:dbl)  [unwired: 1 out]
              n125 = In Range and Coerce(upper limit=0.0, x=w705, lower limit=-inf) -> (coerced(x)=w710:dbl)  [unwired: 1 out]
              n126 = Add(x=w700, y=w699) -> (x+y=w689:dbl)
              n127 = Add(x=w713, y=w701) -> (x+y=w702:dbl)
              n128 = Add(x=w717, y=w710) -> (x+y=w685:dbl)
              n129 = case shown="False" FALSE ("Boolean") {
                tunnel: w749 -> [_ w782]
                tunnel: w748 -> [_ w781]
                tunnel: w747 -> [_ w780]
                tunnel: w746 -> [_ w779]
                tunnel: w745 -> [w765 w778]
                tunnel: [w758 w774] -> w714
                tunnel: w705 -> [w750 w773]
                tunnel: w704 -> [w753 w772]
                tunnel: w703 -> [w760 w771]
                tunnel: w702 -> [w759 w770]
                tunnel: [w755 w769] -> w690
                tunnel: [w754 w768] -> w686
                tunnel: w689 -> [w752 w767]
                tunnel: w685 -> [w751 w766]
                tunnel: w695 -> [w764 _]
                tunnel: w694 -> [w763 _]
                tunnel: w693 -> [w762 _]
                frame False {
                  n130 = Index Array(array=w765, index (dim 0)=w764, index (dim 1)=w762) -> (element=w761:u16[])  [unwired: 1 in]
                  n131 = Index Array(array=w765, index (dim 0)=w764, index (dim 2)=w763) -> (element=w757:u16[])  [unwired: 1 in]
                  n132 = Index Array(array=w765, index (dim 1)=w762, index (dim 2)=w763) -> (element=w756:u16[])  [unwired: 1 in]
                  n133 = Array Subset(array=w757, index=w753, length=w752) -> (w755:u16[])
                  n134 = Array Subset(array=w756, index=w750, length=w751) -> (w754:u16[])
                  n135 = Array Subset(array=w761, index=w760, length=w759) -> (w758:u16[])
                }
                frame True {
                  n136 = Array Subset(array=w778, index (dim 0)=w781, length (dim 0)=w782, index (dim 1)=w780, length (dim 1)=w782, index (dim 2)=w771, length (dim 2)=w770) -> (w777:u16[][][])
                  n137 = Array Subset(array=w778, index (dim 0)=w781, length (dim 0)=w782, index (dim 1)=w772, length (dim 1)=w767, index (dim 2)=w779, length (dim 2)=w782) -> (w775:u16[][][])
                  n138 = Array Subset(array=w778, index (dim 0)=w773, length (dim 0)=w766, index (dim 1)=w780, length (dim 1)=w782, index (dim 2)=w779, length (dim 2)=w782) -> (w776:u16[][][])
                  n139 = for {
                    N: w770 -> [_]
                    tunnel: w777 -> [w792]
                    tunnel: [w790] -> w774 mode=indexing
                    i -> [w789]
                    n140 = Index Array(array=w792, index (dim 2)=w789) -> (element=w791:u16[][])  [unwired: 2 in]
                    n141 = Add Array Elements(numeric array=w791) -> (sum=w790:u16)
                  }
                  n142 = for {
                    N: w766 -> [_]
                    tunnel: [w784] -> w768 mode=indexing
                    tunnel: w776 -> [w783] mode=indexing
                    n143 = Add Array Elements(numeric array=w783) -> (sum=w784:u16)
                  }
                  n144 = for {
                    N: w767 -> [_]
                    tunnel: w775 -> [w788]
                    tunnel: [w786] -> w769 mode=indexing
                    i -> [w785]
                    n145 = Index Array(array=w788, index (dim 1)=w785) -> (element=w787:u16[][])  [unwired: 2 in]
                    n146 = Add Array Elements(numeric array=w787) -> (sum=w786:u16)
                  }
                }
              }
              n147 = call "Gauss fit (SubVI).vi"("parameter bounds"=w731, "Array"=w686, "initial offset"=100.0) -> ("results (a,c,s,r)"=w664:dbl[], "Best Gaussian Fit"=w680:dbl[], "FWHM"=w740:dbl)  [unwired: 2 in, 4 out]
              n148 = call "Gauss fit (SubVI).vi"("parameter bounds"=w731, "Array"=w690, "initial offset"=100.0) -> ("results (a,c,s,r)"=w681:dbl[], "Best Gaussian Fit"=w743:dbl[], "FWHM"=w741:dbl)  [unwired: 2 in, 4 out]
              n149 = call "Gauss fit (SubVI).vi"("parameter bounds"=w731, "Array"=w714, "initial offset"=100.0) -> ("results (a,c,s,r)"=w682:dbl[], "Best Gaussian Fit"=w744:dbl[], "FWHM"=w742:dbl)  [unwired: 2 in, 4 out]
              n150 = local read "pixsize@spl [um]"() -> (w739:dbl)
              n151 = Build Array(w743, w690) -> (w737:dbl[][])
              n152 = Build Array(w680, w686) -> (w736:dbl[][])
              n153 = Build Array(w744, w714) -> (w738:dbl[][])
              n154 = call "Untitled 5 (SubVI).vi"("pixsize"=w684, "results (amplitude,center,stdv,residue,ofst)"=w681, "Array in"=w690) -> ("fit y"=w676:dbl[], "fit x"=w677:dbl[], "real y"=w691:dbl[], "real x"=w692:dbl[])  [unwired: 5 in]
              n155 = call "Untitled 5 (SubVI).vi"("pixsize"=w684, "results (amplitude,center,stdv,residue,ofst)"=w682, "Array in"=w714) -> ("fit y"=w678:dbl[], "fit x"=w679:dbl[], "real y"=w715:dbl[], "real x"=w716:dbl[])  [unwired: 5 in]
              n156 = call "Untitled 5 (SubVI).vi"("pixsize"=w684, "results (amplitude,center,stdv,residue,ofst)"=w664, "Array in"=w686) -> ("fit y"=w674:dbl[], "fit x"=w675:dbl[], "real y"=w687:dbl[], "real x"=w688:dbl[])  [unwired: 5 in]
              n157 = Multiply(x=w741, y=w739) -> (x*y=w734:dbl)
              n158 = Multiply(x=w739, y=w742) -> (x*y=w735:dbl)
              n159 = Multiply(x=w739, y=w740) -> (x*y=w733:dbl)
              n160 = Bundle("real x"=w716, "real y"=w715) -> (w673:cluster{"real x":dbl[], "real y":dbl[]})  [unwired: 1 in]
              n161 = Bundle("fit x"=w679, "fit y"=w678) -> (w672:cluster{"fit x":dbl[], "fit y":dbl[]})  [unwired: 1 in]
              n162 = Bundle("real x"=w692, "real y"=w691) -> (w671:cluster{"real x":dbl[], "real y":dbl[]})  [unwired: 1 in]
              n163 = Bundle("fit x"=w675, "fit y"=w674) -> (w668:cluster{"fit x":dbl[], "fit y":dbl[]})  [unwired: 1 in]
              n164 = Bundle("real x"=w688, "real y"=w687) -> (w669:cluster{"real x":dbl[], "real y":dbl[]})  [unwired: 1 in]
              n165 = Bundle("fit x"=w677, "fit y"=w676) -> (w670:cluster{"fit x":dbl[], "fit y":dbl[]})  [unwired: 1 in]
              n166 = Build Array(w673, w672) -> (w667:cluster{"fit x":dbl[], "fit y":dbl[]}[])
              n167 = Build Array(w671, w670) -> (w666:cluster{"fit x":dbl[], "fit y":dbl[]}[])
              n168 = Build Array(w669, w668) -> (w665:cluster{"fit x":dbl[], "fit y":dbl[]}[])
              n169 = Index Array(array=w681, index #1=w730, index #2=w727) -> (element #1=w724:dbl, element #2=w723:dbl)
              n170 = Index Array(array=w682, index #1=w730, index #2=w727) -> (element #1=w726:dbl, element #2=w725:dbl)
              n171 = Index Array(array=w664, index #1=w730, index #2=w727) -> (element #1=w722:dbl, element #2=w721:dbl)
              n172 = Divide(x=w722, y=w721) -> (x/y=w718:dbl)
              n173 = Divide(x=w724, y=w723) -> (x/y=w719:dbl)
              n174 = Divide(x=w726, y=w725) -> (x/y=w720:dbl)
              n175 = Build Array(w720, w719, w718) -> (w729:dbl[])
              n176 = Array Max & Min(array=w729) -> (max value=w728:dbl)  [unwired: 3 out]
            }
            frame "2D tilted Gaussian fit for zx" {
              w816 = T7 7 items=["Grayscale (U8)", "Grayscale (I16)", "Grayscale (SGL)", "Complex (CSG)", "RGB (U32)", "HSL (U32)", "RGB (U64)", "Grayscale (U16)"] ("Image Type")
              w817 = T7 7 items=["Grayscale (U8)", "Grayscale (I16)", "Grayscale (SGL)", "Complex (CSG)", "RGB (U32)", "HSL (U32)", "RGB (U64)", "Grayscale (U16)"] ("Image Type")
              w848 = 2.0 ("element")
              # "ｘｚで傾いたガウシアンを仮定してフィッティング"
              n177 = Array Subset(array=w867, index (dim 0)=w841, length (dim 0)=w857, index (dim 1)=w869, length (dim 1)=w873, index (dim 2)=w872, length (dim 2)=w857) -> (w866:u16[][][])
              n178 = Array Subset(array=w867, index (dim 0)=w871, length (dim 0)=w873, index (dim 1)=w870, length (dim 1)=w857, index (dim 2)=w868, length (dim 2)=w873) -> (w865:u16[][][])
              n179 = Index Array(array=w866, index (dim 1)=0 ("disabled index (row)")) -> (element=w818:u16[][])  [unwired: 2 in]
              "yx 2" <- w818
              n180 = for {
                N: w857 -> [_]
                tunnel: w865 -> [w878]
                tunnel: [w876] -> w863 mode=indexing
                i -> [w875]
                n181 = Index Array(array=w878, index (dim 1)=w875) -> (element=w877:u16[][])  [unwired: 2 in]
                n182 = Add Array Elements(numeric array=w877) -> (sum=w876:u16)
              }
              n183 = for {
                tunnel: w818 -> [w874] mode=indexing
                tunnel: [w874] -> w852 mode=concatenating
              }
              n184 = Array Max & Min(array=w818) -> (max index (indices)=w833:i32[])  [unwired: 3 out]
              n185 = Array Size(array=w818) -> (size(s)=w838:i32[])
              n186 = call "Gauss fit (SubVI).vi"("parameter bounds"=w846, "Array"=w863) -> ("Best Gaussian Fit"=w864:dbl[], "FWHM"=w862:dbl)  [unwired: 3 in, 5 out]
              n187 = Index Array(array=w833) -> (element #1=w836:i32, element #2=w837:i32)  [unwired: 2 in]
              n188 = Build Array(w864, w863) -> (w844:dbl[][])
              n189 = Build Array(1000.0 ("element"), 0.0 ("element"), w837, w848, w836, w848, 100.0 ("element")) -> (w845:dbl[])
              n190 = call "IMAQ Create"("Image Name"="real", "Image Type"=w817) -> ("New Image"=w826:T1)  [unwired: 3 in, 1 out]
              n191 = call "IMAQ Create"("Image Name"="fit", "Image Type"=w816) -> ("New Image"=w812:T1, "error out"=w811:errorcluster)  [unwired: 3 in]
              n192 = vi-ref "2D tilted Gaussian model.vi"() -> (w856:refnum<vi>)
              n193 = call "IMAQ ArrayToImage"("Image Pixels (U16)"=w818, "Image"=w826) -> ("error out"=w825:errorcluster, "Image Out"=w824:T1)  [unwired: 8 in]
              n194 = call-poly <vilib>:"Nonlinear Curve Fit.vi"("Y"=w852, "f(x,a)"=w856, "X"=w838, "initial parameters"=w845, "termination"=cluster{"max iteration":i32, "tolerance":dbl} {"max iteration"=1000, "tolerance"=1e-08}) -> ("number of function calls"=→"#function calls":i32, "best nonlinear fit"=w843:dbl[], "best fit parameters"=w847:dbl[], "residue"=→"residue":dbl)  [unwired: 3 in, 4 out]
              n195 = Index Array(array=w838) -> (element #1=w840:i32, element #2=w839:i32)  [unwired: 2 in]
              n196 = Reshape Array(w843, w840, w839) -> (w813:dbl[][])
              "yx 3" <- w813
              n197 = call "IMAQ ArrayToImage"("Image Pixels (U16)"=w813, "error in (no error)"=w811, "Image"=w812) -> ("error out"=w814:errorcluster, "Image Out"=w810:T1)  [unwired: 7 in]
              n198 = Index Array(array=w847) -> (element #2=w821:dbl, element #4=w835:dbl, element #6=w834:dbl)  [unwired: 7 in, 4 out]
              n199 = Natural Logarithm(1:2.0 ("x")) -> (0:w831:dbl)
              n200 = Multiply(x=w831, y=8.0) -> (x*y=w829:dbl)
              n201 = local read "pixsize@spl [um]"() -> (w861:dbl)
              n202 = Square Root(x=w829) -> (sqrt(x)=w828:dbl)
              n203 = Compound Arithmetic op=MULTIPLY(w821, invert 3.141592653589793, 180.0 ("value")) -> (w808:dbl)
              "tilt 3" <- w808
              n204 = call "IMAQ Rotate"("error in (no error)"=w825, "Angle (degrees)"=w808, "Image Src"=w824) -> ("error out"=w820:errorcluster, "Image Dst Out"=w819:T1)  [unwired: 7 in]
              n205 = call "IMAQ Rotate"("error in (no error)"=w814, "Angle (degrees)"=w808, "Image Src"=w810) -> ("error out"=w815:errorcluster, "Image Dst Out"=w809:T1)  [unwired: 7 in]
              n206 = call "IMAQ ImageToArray"("error in (no error)"=w820, "Image"=w819) -> ("Image Pixels (U16)"=w799:u16[][])  [unwired: 2 in, 4 out]
              "yx 4" <- w799
              n207 = call "IMAQ ImageToArray"("error in (no error)"=w815, "Image"=w809) -> ("Image Pixels (U16)"=w804:u16[][])  [unwired: 2 in, 4 out]
              "yx 5" <- w804
              n208 = Array Max & Min(array=w799) -> (max index (indices)=w800:i32[])  [unwired: 3 out]
              n209 = Array Max & Min(array=w804) -> (max index (indices)=w806:i32[])  [unwired: 3 out]
              n210 = Index Array(array=w800) -> (element #1=w801:i32, element #2=w802:i32)  [unwired: 2 in]
              n211 = Index Array(array=w806) -> (element #1=w805:i32, element #2=w803:i32)  [unwired: 2 in]
              n212 = Index Array(array=w799, index (row)=w801) -> (element=w797:u16[])  [unwired: 1 in]
              n213 = Index Array(array=w799, index (col)=w802) -> (element=w796:u16[])  [unwired: 1 in]
              n214 = Multiply(x=w862, y=w861) -> (x*y=w859:dbl)
              n215 = Index Array(array=w804, index (row)=w805) -> (element=w798:u16[])  [unwired: 1 in]
              n216 = Index Array(array=w804, index (col)=w803) -> (element=w795:u16[])  [unwired: 1 in]
              n217 = Compound Arithmetic op=MULTIPLY(w861, w835, w828) -> (w860:dbl)
              n218 = Compound Arithmetic op=MULTIPLY(w861, w834, w828) -> (w858:dbl)
              n219 = Build Array(w797, w798) -> (w794:u16[][])
              n220 = Build Array(w796, w795) -> (w793:u16[][])
            }
          }
          n221 = Bundle By Name(cluster=T13 {"x profile"=[], "y profile"=[], "z profile"=[], "FWHMx[um]"=0.0, "FWHMy[um]"=0.0, "FWHMz[um]"=0.0, "z pos"=0, "tilt"=0.0, "error x"=0.0, "error y"=0.0, "error z"=0.0, "error max"=0.0, "coeffs x"=[375.1262519235072, 15.692898037016759, 2.741983029822066, 316.1979872885655, 113.96523182291966], "coeffs y"=[375.1262519235072, 15.692898037016759, 2.741983029822066, 316.1979872885655, 113.96523182291966], "coeffs z"=[375.1262519235072, 15.692898037016759, 2.741983029822066, 316.1979872885655, 113.96523182291966], "profiles x"=[], "profiles y"=[], "profiles z"=[], "x pos"=0, "y pos"=0} ("input cluster"), "x profile"=w651, "y profile"=w650, "z profile"=w649, "FWHMx[um]"=w648, "FWHMy[um]"=w647, "FWHMz[um]"=w646, "z pos"=w609, "tilt"=w644, "error x"=w642, "error y"=w641, "error z"=w640, "error max"=w639, "profiles x"=w608, "coeffs x"=w618, "profiles y"=w607, "coeffs y"=w606, "profiles z"=w605, "coeffs z"=w604, "x pos"=w602, "y pos"=w601) -> (w645:T13)
          "Numeric" <- w643
        }
      }
    }
    n222 = Array Size(array=w347) -> (size(s)=w346:i32)
    n223 = Decrement(x=w346) -> (x-1=w345:i32)
    n224 = property on="raw object index" class="Slide (strict)"("Maximum"=w345, "Minimum"=w344, "Scale.Maximum"=w345, "Scale.Minimum"=w344) -> ()  [unwired: 2 in, 2 out]
    n225 = Index Array(array=w347, index="raw object index") -> (element=w372:i32)
    n226 = local read "Ny"() -> (w464:i32)
    n227 = local read "Nz"() -> (w462:i32)
    n228 = local read "Nx"() -> (w465:i32)
    n229 = Select(t=w366, s="stocked / raw", f=w367) -> (s? t:f=w364:T14)
    n230 = Select(t=w367, s="stocked / raw", f=w366) -> (s? t:f=w365:T14)
    n231 = Multiply(x=w465, y="mag") -> (x*y=w460:dbl)
    n232 = Power Of X(1:2, 2:24) -> (0:w538:dbl)
    n233 = Multiply(x=w464, y="mag") -> (x*y=w459:dbl)
    n234 = Multiply(x=w462, y="mag") -> (x*y=w463:dbl)
    n235 = property on="stocked object index" class="Slide (strict)"("DisabledEnum"=w365) -> ()  [unwired: 2 in, 2 out]
    n236 = property on="raw object index" class="Slide (strict)"("DisabledEnum"=w364) -> ()  [unwired: 2 in, 2 out]
    n237 = property on="add" class="Bool"("DisabledEnum"=w364) -> ()  [unwired: 2 in, 2 out]
    n238 = property on="delete" class="Bool"("DisabledEnum"=w365) -> ()  [unwired: 2 in, 2 out]
    n239 = Decrement(x=w538) -> (x-1=w539:dbl)
    n240 = Select(t=u16 0 ("element"), s="bg black/white", f=w539) -> (s? t:f=w541:dbl)
    n241 = Initialize Array(w541, w459, w460) -> (w537:dbl[][])
    n242 = property on="xz MIP" class="IntGraph (strict)"("Height"=w463, "Width"=w460) -> ()  [unwired: 2 in, 2 out]
    n243 = property on="xy MIP" class="IntGraph (strict)"("Height"=w459, "Width"=w460) -> ()  [unwired: 2 in, 2 out]
    n244 = Bundle(cluster=T12 {"Width"=0, "Height"=0} ("Draw Area Size"), "Width"=w460, "Height"=w459) -> (w542:T12)
    n245 = property on="FWHMx" class="Pict"("Draw Area Size"=w542) -> ()  [unwired: 2 in, 2 out]
    n246 = call-poly <vilib>:"Draw Unflattened Pixmap.vi"("data (RGB format)"=w537) -> ("new picture"=w532:picture)  [unwired: 8 in]
    n247 = for {
      tunnel: "mag" -> [w888]
      tunnel: ["point radius"] -> w546
      shift-right: [w889] -> w545
      shift-left: w532 -> [w891]
      tunnel: w473 -> [w887] mode=indexing
      tunnel: [w886] -> w503 mode=indexing
      tunnel: [w885] -> w513 mode=indexing
      tunnel: [w884] -> w512 mode=indexing
      tunnel: [w883] -> w511 mode=indexing
      tunnel: [w882] -> w491 mode=indexing
      n248 = Unbundle By Name(w887) -> ("x pos"=w880:i32, "y pos"=w881:i32, "FWHMx[um]"=w886:dbl, "FWHMy[um]"=w885:dbl, "FWHMz[um]"=w884:dbl, "z pos"=w883:i32, "error max"=w882:dbl)
      n249 = Multiply(x=w888, y=w880) -> (x*y=w898:dbl)
      n250 = Multiply(x=w881, y=w888) -> (x*y=w897:dbl)
      n251 = Bundle(cluster="pixel center", "horizontal"=w898, "vertical"=w897) -> (w894:cluster{"horizontal":i16, "vertical":i16})
      n252 = call "create color value.vi"("color"="color", "input value"=w886) -> ("color value"=w895:u32)  [unwired: 1 in]
      n253 = call <vilib>:"Draw Circle by Radius.vi"("color(black)"=w895, "fill?(F)"=TRUE, "pixel center"=w894, "radius"="point radius", "picture"=w891) -> ("new picture"=w889:picture)  [unwired: 6 in]
    }
    n254 = Divide(x="plot range", y=2.0) -> (x/y=w527:dbl)
    n255 = local read "mag"() -> (w558:dbl)
    n256 = Array Size(array=w503) -> (size(s)=w502:i32)
    n257 = Array Size(array=w454) -> (size(s)=w453:i32[])
    n258 = call "sort 1D array with index (SubVI).vi"("input"=w513) -> ("indices"=w509:i32[])  [unwired: 9 in, 1 out]
    n259 = call "sort 1D array with index (SubVI).vi"("input"=w503) -> ("indices"=w510:i32[])  [unwired: 9 in, 1 out]
    n260 = call "sort 1D array with index (SubVI).vi"("input"=w512) -> ("indices"=w508:i32[])  [unwired: 9 in, 1 out]
    n261 = call "sort 1D array with index (SubVI).vi"("input"=w511) -> ("indices"=w507:i32[])  [unwired: 9 in, 1 out]
    n262 = call "sort 1D array with index (SubVI).vi"("input"=w491) -> ("indices"=w490:i32[])  [unwired: 9 in, 1 out]
    n263 = local read "z ofst and pixsize"() -> (w458:dbl[])
    n264 = Add(x=i16 4, y=w546) -> (x+y=w548:i16)
    n265 = for {
      N: w502 -> [_]
      tunnel: [w879] -> w501 mode=indexing
      i -> [w879]
    }
    n266 = Index Array(array=w453) -> (element=w450:i32)  [unwired: 1 in]
    n267 = call <vilib>:"Histogram.vi"("intervals"="intervals", "X"=w512) -> ("Histogram Graph"=→"FWHMz":T4)  [unwired: 6 in, 3 out]
    n268 = call <vilib>:"Histogram.vi"("intervals"="intervals", "X"=w503) -> ("Histogram Graph"=→"FWHMx":T4)  [unwired: 6 in, 3 out]
    n269 = call <vilib>:"Histogram.vi"("intervals"="intervals", "X"=w513) -> ("Histogram Graph"=→"FWHMy":T4)  [unwired: 6 in, 3 out]
    n270 = Array Max & Min(array=w503) -> (max value=→"max":dbl, min value=→"min":dbl)  [unwired: 2 out]
    n271 = Divide(x=w450, y=2) -> (x/y=w448:dbl)
    n272 = Build Array(w501, w510, w509, w508, w507, w490) -> (w506:i32[][])
    n273 = Index Array(array=w458) -> (element #1=w456:dbl, element #2=w455:dbl)  [unwired: 2 in]
    n274 = Negate(x=w456) -> (-x=w342:dbl)
    n275 = Index Array(array=w506, index (row)="indexing variable") -> (element=w504:i32[])  [unwired: 1 in]
    n276 = call "IMAQ Create"("Image Name"="zx", "Image Type"=w438) -> ("New Image"=w436:T1, "error out"=w440:errorcluster)  [unwired: 3 in]
    n277 = local read "file path (use dialog)"() -> (w489:path)
    n278 = call "color config.vi"("color 1"="color 3") -> ("Array"=w495:cluster{dbl, u32}[])  [unwired: 9 in, 1 out]
    n279 = property on="xy MIP" class="IntGraph (strict)"("ZScale.MarkerVals[]"=w495) -> ()  [unwired: 2 in, 2 out]
    n280 = property on="xz MIP" class="IntGraph (strict)"("ZScale.MarkerVals[]"=w495) -> ()  [unwired: 2 in, 2 out]
    n281 = Path To String(path=w489) -> (string=w467:string)
    n282 = Multiply(x="nx'", y=2) -> (x*y=w417:i32)
    n283 = Multiply(x="nz'", y=2) -> (x*y=w420:i32)
    n284 = Increment(x=w417) -> (x+1=w412:i32)
    n285 = Increment(x=w420) -> (x+1=w419:i32)
    n286 = call "color config.vi"("color 1"="color 2") -> ("Array"=w383:cluster{dbl, u32}[])  [unwired: 9 in, 1 out]
    n287 = local read "parameter bounds 2"() -> (w343:T5)
    n288 = property on="yx" class="IntGraph (strict)"("ZScale.MarkerVals[]"=w383) -> ()  [unwired: 2 in, 2 out]
    n289 = property on="zx" class="IntGraph (strict)"("ZScale.MarkerVals[]"=w383) -> ()  [unwired: 2 in, 2 out]
    n290 = property on="zx 2" class="IntGraph (strict)"("ZScale.MarkerVals[]"=w383) -> ()  [unwired: 2 in, 2 out]
    n291 = property on="zy" class="IntGraph (strict)"("ZScale.MarkerVals[]"=w383) -> ()  [unwired: 2 in, 2 out]
    n292 = local read "pixsize@spl [um]"() -> (w397:dbl)
    n293 = feedback #2(T10 []) -> (w378:T10)
    n294 = feedback #3(i32[] []) -> (w353:i32[])
    n295 = Index Array(array=w353, index="stocked object index") -> (element=w371:i32)
    n296 = Array Size(array=w353) -> (size(s)=w355:i32)
    "num of points" <- w355
    n297 = Decrement(x=w355) -> (x-1=w357:i32)
    n298 = property on="stocked object index" class="Slide (strict)"("Maximum"=w357, "Minimum"=0.0 ("Data Entry Limits:Minimum"), "Scale.Maximum"=w357, "Scale.Minimum"=0.0 ("Scale.Range:Minimum")) -> ()  [unwired: 2 in, 2 out]
    n299 = Select(t=w372, s="stocked / raw", f=w371) -> (s? t:f=w369:i32)
    "obj index" <- w369
    n300 = Index Array(array=w466, index=w369) -> (element=w471:T16)
    n301 = Index Array(array=w473, index=w369) -> (element=w470:T13)
    n302 = Unbundle(w470) -> ("x profile"=→"x2":dbl[][], "y profile"=→"y2":dbl[][], "z profile"=→"z2":dbl[][], "FWHMx[um]"=→"FWHMx [um]":dbl, "FWHMy[um]"=→"FWHMy [um]":dbl, "FWHMz[um]"=→"FWHMz [um]":dbl, "z pos"=w452:i32, "tilt"=w500:dbl, "error x"=→"error x":dbl, "error y"=→"error y":dbl, "error z"=→"error z":dbl, "profiles x"=→"x":cluster{dbl[], dbl[]}[], "profiles y"=→"y":cluster{dbl[], dbl[]}[], "profiles z"=→"z":cluster{dbl[], dbl[]}[], "x pos"=w341:i32, "y pos"=w340:i32)  [unwired: 4 out]
    "Y" <- w340
    "X" <- w341
    "Z" <- w452
    n303 = Compound Arithmetic op=MULTIPLY(w500, invert 3.141592653589793, -180.0 ("value")) -> (→"tilt 2":dbl)
    n304 = Subtract(x=w452, y=w527) -> (x-y=w526:dbl)
    n305 = Subtract(x=w340, y=w527) -> (x-y=w524:dbl)
    n306 = Subtract(x=w341, y=w527) -> (x-y=w525:dbl)
    n307 = Index Array(array=w454, index (dim 1)=w340) -> (element=w530:u16[][])  [unwired: 2 in]
    n308 = Index Array(array=w454, index (dim 2)=w341) -> (element=w529:u16[][])  [unwired: 2 in]
    n309 = Index Array(array=w454, index (dim 0)=w452) -> (element=w531:u16[][])  [unwired: 2 in]
    n310 = Multiply(x=w558, y=w340) -> (x*y=w555:dbl)
    n311 = Multiply(x=w558, y=w341) -> (x*y=w554:dbl)
    n312 = Bundle(cluster=cluster{"horizontal":i16, "vertical":i16} {"horizontal"=45, "vertical"=45} ("pixel center 2"), "horizontal"=w554, "vertical"=w555) -> (w557:cluster{"horizontal":i16, "vertical":i16})
    n313 = Array Subset(array=w530, index (row)=w526, length (row)="plot range", index (col)=w525, length (col)="plot range") -> (w437:u16[][])
    "zx" <- w437
    n314 = Array Subset(array=w529, index (row)=w526, length (row)="plot range", index (col)=w524, length (col)="plot range") -> (w468:u16[][])
    "zy" <- w468
    n315 = Array Subset(array=w531, index (row)=w524, length (row)="plot range", index (col)=w525, length (col)="plot range") -> (w469:u16[][])
    "yx" <- w469
    n316 = call <vilib>:"Draw Circle by Radius.vi"("pen"=T11 {"Width"=2, "Style"=enum."Solid"} ("marker pen"), "color(black)"="marker", "pixel center"=w557, "radius"=w548, "picture"=w545) -> ("new picture"=→"FWHMx":picture)  [unwired: 6 in]
    n317 = Subtract(x=w452, y=w448) -> (x-y=w451:dbl)
    n318 = Multiply(x=w455, y=w451) -> (x*y=w457:dbl)
    n319 = Subtract(x=w342, y=w457) -> (x-y=w338:dbl)
    "z [um]" <- w338
    n320 = call "IMAQ ArrayToImage"("Image Pixels (U16)"=w437, "error in (no error)"=w440, "Image"=w436) -> ("error out"=w435:errorcluster, "Image Out"=w434:T1)  [unwired: 7 in]
    n321 = call "IMAQ Rotate 2"("Interpolation Type"=w431, "Maintain Size"=TRUE, "error in (no error)"=w435, "Angle (degrees)"="Angle (degrees)", "Image Src"=w434) -> ("error out"=w430:errorcluster, "Image Dst Out"=w428:T1)  [unwired: 5 in]
    n322 = Select(t=w338, s="save z pos?", f="saved parameter") -> (s? t:f=w336:dbl)
    n323 = call "IMAQ ImageToArray"("error in (no error)"=w430, "Image"=w428) -> ("Image Pixels (U16)"=w426:u16[][], "error out"=w429:errorcluster)  [unwired: 2 in, 3 out]
    "zx 2" <- w426
    n324 = Array Max & Min(array=w426) -> (max index (indices)=w427:i32[])  [unwired: 3 out]
    n325 = call "IMAQ Dispose"("Image"=w428, "error in (no error)"=w429) -> ("error out"=w439:errorcluster)  [unwired: 4 in]
    n326 = Index Array(array=w427) -> (element #1=w423:i32, element #2=w414:i32)  [unwired: 2 in]
    n327 = call <vilib>:"Simple Error Handler.vi"("error in (no error)"=w439) -> ()  [unwired: 4 in, 5 out]
    n328 = Index Array(array=w426, index (col)=w414) -> (element=w424:u16[])  [unwired: 1 in]
    n329 = Index Array(array=w426, index (row)=w423) -> (element=w425:u16[])  [unwired: 1 in]
    n330 = Subtract(x=w423, y="nz'") -> (x-y=w418:i32)
    n331 = Subtract(x=w414, y="nx'") -> (x-y=w413:i32)
    n332 = Array Subset(array=w425, index=w413, length=w412) -> (w403:u16[])
    n333 = Array Subset(array=w424, index=w418, length=w419) -> (w399:u16[])
    n334 = call "Gauss fit (SubVI).vi"("parameter bounds"=w343, "Array"=w403, "initial offset"=100.0) -> ("results (a,c,s,r)"=w402:dbl[], "FWHM"=w409:dbl)  [unwired: 2 in, 5 out]
    n335 = call "Gauss fit (SubVI).vi"("parameter bounds"=w343, "Array"=w399, "initial offset"=100.0) -> ("results (a,c,s,r)"=w398:dbl[], "FWHM"=w408:dbl)  [unwired: 2 in, 5 out]
    n336 = Multiply(x=w397, y=w409) -> (x*y=w390:dbl)
    "FWHMx'" <- w390
    n337 = Multiply(x=w397, y=w408) -> (x*y=w389:dbl)
    "FWHMz'" <- w389
    n338 = call "Untitled 5 (SubVI).vi"("pixsize"=w397, "results (amplitude,center,stdv,residue,ofst)"=w402, "Array in"=w403) -> ("fit y"=w407:dbl[], "fit x"=w406:dbl[], "real y"=w405:dbl[], "real x"=w404:dbl[])  [unwired: 5 in]
    n339 = call "Untitled 5 (SubVI).vi"("pixsize"=w397, "results (amplitude,center,stdv,residue,ofst)"=w398, "Array in"=w399) -> ("fit y"=w395:dbl[], "fit x"=w396:dbl[], "real y"=w400:dbl[], "real x"=w401:dbl[])  [unwired: 5 in]
    n340 = Bundle("real x"=w404, "real y"=w405) -> (w394:cluster{"real x":dbl[], "real y":dbl[]})  [unwired: 1 in]
    n341 = Bundle("fit x"=w406, "fit y"=w407) -> (w393:cluster{"fit x":dbl[], "fit y":dbl[]})  [unwired: 1 in]
    n342 = Bundle("fit x"=w396, "fit y"=w395) -> (w391:cluster{"fit x":dbl[], "fit y":dbl[]})  [unwired: 1 in]
    n343 = Bundle("real x"=w401, "real y"=w400) -> (w392:cluster{"real x":dbl[], "real y":dbl[]})  [unwired: 1 in]
    n344 = Build Array(w394, w393) -> (w387:cluster{"fit x":dbl[], "fit y":dbl[]}[])
    "x'" <- w387
    n345 = Build Array(w392, w391) -> (w388:cluster{"fit x":dbl[], "fit y":dbl[]}[])
    "z'" <- w388
    n346 = Bundle By Name(cluster=T9 {"z [um]"=0.0, "Particle Report"={"Area"=0.0, "Number of Holes"=0.0, "Bounding Rect"={"Left"=0.0, "Top"=0.0, "Right"=0.0, "Bottom"=0.0}, "Center of Mass"={"X"=0.0, "Y"=0.0}, "Orientation"=0.0, "Dimensions"={"Width"=0.0, "Height"=0.0}}, "yx"=[], "zx"=[], "zy"=[], "filepath"="", "FWHMx'"=0.0, "x' profiles"=[], "FWHMz'"=0.0, "z' profiles"=[], "input cluster"={"x profile"=[], "y profile"=[], "z profile"=[], "FWHMx[um]"=0.0, "FWHMy[um]"=0.0, "FWHMz[um]"=0.0, "z pos"=0, "tilt"=0.0, "error x"=0.0, "error y"=0.0, "error z"=0.0, "error max"=0.0, "coeffs x"=[375.1262519235072, 15.692898037016759, 2.741983029822066, 316.1979872885655, 113.96523182291966], "coeffs y"=[375.1262519235072, 15.692898037016759, 2.741983029822066, 316.1979872885655, 113.96523182291966], "coeffs z"=[375.1262519235072, 15.692898037016759, 2.741983029822066, 316.1979872885655, 113.96523182291966], "profiles x"=[], "profiles y"=[], "profiles z"=[], "x pos"=0, "y pos"=0}} ("output cluster"), "z [um]"=w336, "Particle Report"=w471, "input cluster"=w470, "yx"=w469, "zx"=w437, "zy"=w468, "filepath"=w467, "FWHMx'"=w390, "x' profiles"=w387, "FWHMz'"=w389, "z' profiles"=w388) -> (w377:T9)
    n347 = for {
      tunnel: w353 -> [w564] mode=indexing
      tunnel: "raw object index" -> [w563]
      shift-right: [w560] -> w349
      shift-left: TRUE -> [w561]
      n348 = Not Equal?(x=w564, y=w563) -> (x != y?=w562:bool)
      n349 = And(x=w562, y=w561) -> (x .and. y?=w560:bool)
    }
    n350 = And(x=w349, y="add") -> (x .and. y?=w350:bool)
    n351 = case shown="True" w350 {
      tunnel: w378 -> [w582 w588]
      tunnel: w377 -> [_ w587]
      tunnel: [w582 w586] -> w376
      tunnel: w353 -> [w581 w585]
      tunnel: [w581 w584] -> w374
      tunnel: "raw object index" -> [_ w583]
      frame False {
      }
      frame True {
        n352 = Insert Into Array(array=w585, new element=w583) -> (w584:i32[])  [unwired: 1 in]
        n353 = Insert Into Array(array=w588, new element=w587) -> (w586:T10)  [unwired: 1 in]
      }
    }
    n354 = case shown="True" "delete" {
      tunnel: [w573 w579] -> w363
      tunnel: w376 -> [w573 w580]
      tunnel: w374 -> [w572 w577]
      tunnel: [w572 w576] -> w373
      tunnel: "stocked object index" -> [_ w574]
      frame False {
      }
      frame True {
        n355 = Delete From Array(array=w580, length=1, index=w574) -> (array with subset deleted=w579:T10)  [unwired: 1 out]
        n356 = Delete From Array(array=w577, length=1, index=w574) -> (array with subset deleted=w576:i32[])  [unwired: 1 out]
      }
    }
    n357 = feedback-in #2(w363) -> ()
    n358 = feedback-in #3(w373) -> ()
    n359 = for {
      tunnel: [w571] -> w382 mode=indexing
      tunnel: [w570] -> w447 mode=indexing
      tunnel: [w569] -> w446 mode=indexing
      tunnel: [w568] -> w445 mode=indexing
      tunnel: [w567] -> w381 mode=indexing
      tunnel: [w566] -> w380 mode=indexing
      tunnel: w363 -> [w565] mode=indexing
      n360 = Unbundle By Name(w565) -> ("z [um]"=w571:dbl, "input cluster.FWHMx[um]"=w570:dbl, "input cluster.FWHMy[um]"=w569:dbl, "input cluster.FWHMz[um]"=w568:dbl, "FWHMx'"=w567:dbl, "FWHMz'"=w566:dbl)
    }
    n361 = Bundle(w382, w380) -> (w359:cluster{dbl[], dbl[]})  [unwired: 1 in]
    n362 = Bundle(w382, w381) -> (w362:cluster{dbl[], dbl[]})  [unwired: 1 in]
    n363 = Bundle(w382, w445) -> (w442:cluster{dbl[], dbl[]})  [unwired: 1 in]
    n364 = Bundle(w382, w447) -> (w444:cluster{dbl[], dbl[]})  [unwired: 1 in]
    n365 = Bundle(w382, w446) -> (w443:cluster{dbl[], dbl[]})  [unwired: 1 in]
    n366 = Build Array(w444, w443, w442, w362, w359) -> (→"profile 2":cluster{dbl[], dbl[]}[])
    "Numeric 2" <- w476
  }
  n367 = Array Size(array=w7) -> (size(s)=w6:i32)
  n368 = Not Equal To 0?(x=w6) -> (x != 0?=w5:bool)
  n369 = Open/Create/Replace File(file path (use dialog)="analysis file", operation (0:open)=T8."open or create") -> (refnum out=w35:refnum<file>, error out=w34:errorcluster)  [unwired: 4 in, 1 out]
  n370 = case shown="True" w5 {
    tunnel: w35 -> [w900 w908]
    tunnel: w34 -> [w899 w907]
    tunnel: [w900 w903] -> w26
    tunnel: [w899 w902] -> w25
    tunnel: w7 -> [_ w901]
    frame False {
    }
    frame True {
      n371 = Set File Position(offset (in bytes) (0)=i64 0, refnum=w908, from (0:start)=enum16{"start", "end", "current"}."end", error in=w907) -> (refnum out=w905:refnum<file>, error out=w904:errorcluster)
      n372 = for {
        tunnel: w901 -> [w914] mode=indexing
        tunnel: w905 -> [w913]
        tunnel: w904 -> [w912]
        tunnel: [w911] -> w903
        tunnel: [w910] -> w902
        n373 = Write to Binary File(file (use dialog)=w913, data=w914, error in=w912) -> (refnum out=w911:refnum<file>, error out=w910:errorcluster)  [unwired: 3 in, 1 out]
      }
    }
  }
  n374 = Set File Position(offset (in bytes) (0)=i64 0, refnum=w26, from (0:start)=enum16{"start", "end", "current"}."start", error in=w25) -> (refnum out=w24:refnum<file>, error out=w22:errorcluster)
  n375 = while {
    tunnel: w24 -> [w923]
    tunnel: w22 -> [w922]
    tunnel: [w921] -> w9 mode=indexing if=w915
    tunnel: [w920] -> w23
    tunnel: [w918] -> _
    tunnel: [w919] -> w8
    i -> [w919]
    stop <- w916 stop-if-true
    n376 = Read from Binary File(5:T9 {"z [um]"=0.0, "Particle Report"={"Area"=0.0, "Number of Holes"=0.0, "Bounding Rect"={"Left"=0.0, "Top"=0.0, "Right"=0.0, "Bottom"=0.0}, "Center of Mass"={"X"=0.0, "Y"=0.0}, "Orientation"=0.0, "Dimensions"={"Width"=0.0, "Height"=0.0}}, "yx"=[], "zx"=[], "zy"=[], "filepath"="", "FWHMx'"=0.0, "x' profiles"=[], "FWHMz'"=0.0, "z' profiles"=[], "input cluster"={"x profile"=[], "y profile"=[], "z profile"=[], "FWHMx[um]"=0.0, "FWHMy[um]"=0.0, "FWHMz[um]"=0.0, "z pos"=0, "tilt"=0.0, "error x"=0.0, "error y"=0.0, "error z"=0.0, "error max"=0.0, "coeffs x"=[375.1262519235072, 15.692898037016759, 2.741983029822066, 316.1979872885655, 113.96523182291966], "coeffs y"=[375.1262519235072, 15.692898037016759, 2.741983029822066, 316.1979872885655, 113.96523182291966], "coeffs z"=[375.1262519235072, 15.692898037016759, 2.741983029822066, 316.1979872885655, 113.96523182291966], "profiles x"=[], "profiles y"=[], "profiles z"=[], "x pos"=0, "y pos"=0}} ("output cluster"), 8:w922, 11:w923) -> (0:w918:errorcluster, 2:w921:T9, 3:w920:refnum<file>)  [unwired: 3 in, 1 out]
    n377 = Unbundle By Name(w918) -> ("status"=w916:bool)
    n378 = Not(x=w916) -> (.not. x?=w915:bool)
  }
  "Numeric 3" <- w8
  n379 = for {
    tunnel: [w930] -> w16 mode=indexing
    tunnel: [w929] -> w10 mode=indexing
    tunnel: [w928] -> w11 mode=indexing
    tunnel: [w927] -> w12 mode=indexing
    tunnel: [w926] -> w17 mode=indexing
    tunnel: [w925] -> w18 mode=indexing
    tunnel: w9 -> [w924] mode=indexing
    n380 = Unbundle By Name(w924) -> ("z [um]"=w930:dbl, "input cluster.FWHMx[um]"=w929:dbl, "input cluster.FWHMy[um]"=w928:dbl, "input cluster.FWHMz[um]"=w927:dbl, "FWHMx'"=w926:dbl, "FWHMz'"=w925:dbl)
  }
  n381 = Bundle(w16, w18) -> (w21:cluster{dbl[], dbl[]})  [unwired: 1 in]
  n382 = Bundle(w16, w17) -> (w19:cluster{dbl[], dbl[]})  [unwired: 1 in]
  n383 = Bundle(w16, w12) -> (w15:cluster{dbl[], dbl[]})  [unwired: 1 in]
  n384 = Bundle(w16, w10) -> (w13:cluster{dbl[], dbl[]})  [unwired: 1 in]
  n385 = Bundle(w16, w11) -> (w14:cluster{dbl[], dbl[]})  [unwired: 1 in]
  n386 = Build Array(w13, w14, w15, w19, w21) -> (→"profile 3":cluster{dbl[], dbl[]}[])
  n387 = Close File(refnum=w23, error in=w22) -> ()  [unwired: 2 out]
